vi "Dashboard Main.vi"() -> ()   [LabVIEW 2020]
uses:
  <vilib>/Utility/miscctls.llb/LVRectTypeDef.ctl
  <vilib>/Utility/miscctls.llb/LVRowAndColumnTypeDef.ctl
  <vilib>/event_ctls.llb/eventvkey.ctl
  <vilib>/Rock Robotics/WPI/DriverStation/WPI_DriverStationAllianceInfo.ctl
  <vilib>/Utility/xml.llb/Read From XML File(array).vi
  <vilib>/Utility/xml.llb/Write to XML File(string).vi
  <vilib>/Rock Robotics/Network Tables/NT Read Boolean.vi
  <vilib>/Rock Robotics/Network Tables/NT Write Boolean.vi
  <vilib>/Rock Robotics/Network Tables/NT Read Boolean Array.vi
  <vilib>/Rock Robotics/Network Tables/NT Write Boolean Array.vi
  <vilib>/Rock Robotics/Network Tables/NT Write Numeric Array.vi
  <vilib>/Rock Robotics/Network Tables/NT Read Numeric Array.vi
  <vilib>/Rock Robotics/WPI/Dashboard/WPI_DashboardLogging Global.vi
  <vilib>/Rock Robotics/Network Tables/NT Write String Array.vi
  <vilib>/vision/NI_Vision_Development_Module.lvlib
panel:
  out "Legal_Drivers":string[](array[string])
  out "Shooter_Motor_Failure_Array":bool[](array[boolean])
  out "Shooter_Overheat_Array":bool[](array[boolean])
  out "Shifter_Faults_Array":bool[](array[boolean])
  out "Drive_Overheat_Array":bool[](array[boolean])
  out "Audible_Warnings_Enabled":bool
  in  "TCP":refnum<k5>
  in  "Rec Mode":enum32{"Stop", "Record", "Playback"}(radio)
  out "Image Message":string="Timeout in Camera Communications"
  in  "Dashboard Tab":T1(tab)=enum."Setup/Auto"
  in  "CheckList":i32(listbox)
  out "Match_End":bool
  out "Auto Playbook Entry":string
  out "Drive Action":string
  out "Manipulator Action":string
  in  "Driver Profile":u16(ring) items=["N/A"]
  in  "Camera Name":string(combo)="limelight"
  in  "Camera Settings":T2={"Frame Rate"=20, "Compression"=60, "Size"=1, "DB Camera Config"=FALSE} {"Size" items=["640x480", "320x240", "160x120"]}
  in  "Autonomous Play":u16(ring) items=["N/A"]
  out "Robot Pose":cluster{dbl[], dbl[]}[](graph)
  out "Master_Caution_0":bool caption="Mode_Butterfly"
  out "Robot_is_Autonomous_0":bool caption="Mode_Butterfly"
  in  "Robot Profile":u16(ring) items=["N/A"]
  out "Robot_Code_Version":string
  in  "Default Camera Pipeline":u16(ring) items=["N/A"]
  out "Auto_Suffix":string
  in  "Refresh_Auto_Play_List":bool
  in  "Auto_Delay":dbl format="%.1f"
  in  "Warning Time (s)":dbl=30.0 format="%.1f"
  in  "Manual_Start_X":dbl=509.25 format="%.1f"
  in  "Disable_Fusion_X":bool=TRUE
  out "Robot X":dbl format="%.1f"
  out "Robot Y":dbl format="%.1f"
  in  "Manual_Start_Y":dbl=94.66 format="%.1f"
  in  "Disable_Fusion_Y":bool=TRUE
  out "Robot H":dbl format="%.1f"
  in  "Manual_Start_H":dbl format="%.1f"
  out "Distance_To_Target_Detail":dbl format="%.1f"
  in  "Field Map":u16(ring) items=["N/A"]
  in  "Push_Robot_Start":bool
  in  "Export_Robot_Pose":bool
  in  "Clear_Robot_Pose_Display":bool
  in  "Dock_Dashboard":bool
  in  "Hide_Popups":bool
  in  "Force_Human_Control":bool
  in  "Auto_Test_Mode":bool
  out "Camera_1_Fault":bool
  out "Pressure_Leak":bool
  in  "Master_Safety_Override_2":bool
  in  "Master_Safety_Override_1":bool
  out "LIDAR_Fault":bool
  out "Help Graphic":T3(plugin-control)
  in  "Manipulator_Help":bool
  out "Cowl_Position":dbl(knob) scale=0.0..1.0
  in  "Driver_Help":bool
  in  "Error_Help":bool
  out "Camera_2_Fault":bool
  out "Robot Pose 1":cluster{dbl[], dbl[]}[](graph)
  out "Drive_Train_Shifter":bool
  out "Electrical_Fault":bool
  out "Diverting_Power":bool
  out "Shooter_Power":dbl(knob) scale=0.0..1.0
  out "Kicker_Power":dbl(knob) scale=0.0..1.0
  out "CAN_Bus_Fault":bool
  out "IMU_Failure":bool
  out "Robot_is_Autonomous_1":bool caption="Mode_Butterfly"
  in  "Pre_Spin":bool
  out "LL_Valid":bool caption="Mode_Butterfly"
  in  "Clear_Jams":bool
  out "Balls_Shot":i32 format="%#.0f"
  out "Ret_Feeder_Left":bool
  out "Ret_Feeder_Right":bool
  out "Tablet_Override":bool
  out "Match Time(s)":sgl format="%#.0f"
  out "Intake_Overheat":bool
  out "Ret_Ball_Left":bool
  out "Ret_Ball_Right":bool
  out "Shooter_Motor_Failure":bool
  out "Intake_On":bool caption="Mode_Butterfly"
  out "Shooter_Overheat":bool
  out "Auto_Error":bool
  in  "Clear_Errors":bool
  out "Drive_Train_Azimuth":bool
  out "Pressure_Transducer":dbl(slide) scale=0.0..120.0
  out "Pressure_Vent":bool
  out "Shooter_RPM_Actual":dbl(slide) scale=0.0..5700.0
  out "Drive_Train_Overheat":bool
  out "Compressor_On":bool
  out "Ret_Power_Port_Right":bool
  out "Ret_Power_Port_Left":bool
  in  "Right":bool
  in  "Reticule":T4(ring)
  in  "Save":bool
  in  "Up":bool
  in  "Down":bool
  in  "Left":bool
  out "Master_Caution_1":bool caption="Mode_Butterfly"
  out "Battery_Critical":bool
  out "Battery_Voltage":dbl(slide) scale=11.0..13.0
  out "Field_Oriented":bool caption="Mode_Butterfly"
  out "Shooter_RPM_Goal":dbl(slide) scale=0.0..5700.0
  out "Slow_Loop":bool
  in  "Mode_TargetingComputer":bool
  in  "Mode_Wall":bool
  in  "Arm_Climber":bool
  in  "State_Normal":bool
  in  "State_Rotation_Control":bool
  in  "State_Climb":bool
  in  "Mode_InitiationLine":bool
  in  "Mode_CloseTrench":bool
  in  "Mode_FarTrench":bool
  in  "State_Position_Control":bool
  out "Combined Camera Feed":T3(plugin-control)
  out "High_Gear_0":bool
  out "High_Gear_1":bool
  out "High_Gear_2":bool
  out "High_Gear_3":bool
  out "Pointed_At_Target":bool caption="Mode_Butterfly"
  out "Shooter_Ready":bool caption="Mode_Butterfly"
  out "Shooter_Firing":bool caption="Mode_Butterfly"
  out "Shooter_Spinning":bool caption="Mode_Butterfly"
  out "Climber_Climbing":bool caption="Mode_Butterfly"
  out "Shooter_1_Temp":dbl
  out "Shooter_RPM_Goal_Detail":dbl
  out "Wheel_3S_Velocity":dbl format="%.1f"
  out "Wheel_3_Azimuth":dbl format="%.1f"
  out "Wheel_3S_Temp":dbl
  out "Wheel_0S_Temp":dbl
  in  "Select Auto":string(combo)="Select Autonomous ..."
  out "Camera Perf":string
  out "Control Loop Time (ms)":u32
  in  "Calibrate_Wheels":bool
  in  "Zero_Wheels":bool
  out "Wheel_0_Azimuth":dbl format="%.1f"
  out "Wheel_0S_Velocity":dbl format="%.1f"
  out "Wheel_1S_Velocity":dbl format="%.1f"
  out "Wheel_1_Azimuth":dbl format="%.1f"
  out "Wheel_1S_Temp":dbl
  out "Wheel_2S_Velocity":dbl format="%.1f"
  out "Wheel_2_Azimuth":dbl format="%.1f"
  out "Wheel_2S_Temp":dbl
  in  "Arm_Calibrate":bool
  out "Shooter_0_RPM_Actual_Detail":dbl
  out "Master_Caution_2":bool caption="Mode_Butterfly"
  out "Shooter_0_Temp":dbl
  out "Shooter_1_RPM_Actual_Detail":dbl
  out "Out_Of_Range":bool
  in  "New_Shooter_Setpoint (rpm)":dbl=3000.0 min=0.0 max=5700.0 step=100.0
  out "Kicker_RPM_Actual_Detail":dbl
  out "Kicker_RPM_Goal_Detail":dbl
  out "Kicker_Temp":dbl
  out "Intake_Temp":dbl
  in  "Actuator Testing":u16(ring) items=["N/A"]
  in  "Test_Actuator_Value":dbl step=0.1 format="%.2f"
  in  "Calibrate_Joysticks":bool
  in  "Arm_Calibrate_Joysticks":bool
  out "Robot_is_Autonomous_2":bool caption="Mode_Butterfly"
  in  "Test_Actuator_Period":dbl min=0.0 step=1.0 format="%.2f"
  out "Pose Loop Time (ms)":u32
  in  "Mute_Audible_Warnings":bool
  out "Combined Error String":string
  out "LIDAR_Distance_To_Target":dbl format="%.1f"
  out "Beam_Break_Raw":i32
  out "Wheel_0_Shifter_State":string
  out "Wheel_1_Shifter_State":string
  out "Wheel_3_Shifter_State":string
  out "Wheel_2_Shifter_State":string
  out "Azimuth_Error_Array":bool[](array[boolean])
  out "Selected_Shooter_Setpoint_Value (rpm)":dbl
  in  "Apply_New_Shooter_Setpoint":bool
  in  "Selected_Shooter_Setpoint_Index":u16(ring) items=["N/A"]
  in  "Auto_Target_Override":bool
  in  "Field_Oriented_Override":bool
  in  "Camera_Override":bool
  in  "Super_Test_Mode":bool
  out "Current_Driver_Profile_Setpoints":T5={"Strafe Deadband"=0.08, "Strafe Scaling"=2.0, "Strafe Maximum"=0.5, "Rotation Deadband"=0.15, "Rotation Scaling"=2.5, "Rotation Maximum"=0.5} {"Rotation Maximum" min=0.3 max=1.0 scale=0.3..1.0; "Rotation Scaling" min=1.0 max=4.0 scale=1.0..4.0; "Rotation Deadband" min=0.0 max=0.25 scale=0.0..0.25; "Strafe Maximum" min=0.3 max=1.0 scale=0.3..1.0; "Strafe Scaling" min=1.0 max=4.0 scale=1.0..4.0; "Strafe Deadband" min=0.0 max=0.25 scale=0.0..0.25}
  in  "New_Driver_Profile_Setpoints":T6={"Strafe Deadband"=0.08, "Strafe Scaling"=2.0, "Strafe Max"=0.5, "Rotate Deadband"=0.15, "Rotate Scaling"=2.5, "Rotate Max"=0.5} {"Rotate Max" min=0.3 max=1.0 format="%.2g"; "Rotate Scaling" min=1.0 max=4.0 format="%.2g"; "Rotate Deadband" min=0.0 max=0.25 format="%.2g"; "Strafe Max" min=0.3 max=1.0 format="%.2g"; "Strafe Scaling" min=1.0 max=4.0 format="%.2g"; "Strafe Deadband" min=0.0 max=0.25 format="%.2g"}
  in  "Apply_Driver_Profile_Setpoints":bool
  out "Current_Driver_Profile":string
  out "NT Connection":bool
  out "Mode":T7(ring)=enum."Auto Disabled"
  in  "Test Slider":dbl(slide) scale=0.0..100.0 scale format="%#_3g"
  in  "On/Off":bool caption="Solenoid"
  in  "Test Name":u16(ring) items=["Select the test to run..."]
  in  "Test Tree":string(tree)
  in  "Motor":cluster{"Value":dbl, "Enable":bool} {"Value" scale=-1.0..1.0 scale format="%#_3g"}
  out "Progress":T8 {"Test Progress" scale=0.0..100.0}
  in  "Rev/Fwd":cluster{"Forward":bool, "Reverse":bool}
  in  "Test Ring":u16(ring) items=["Monochrome", "Color"]
  out "Cmd Status":string
  in  "Execute Command":bool
  in  "Command Params":string[][](table)
  in  "Command Selection":i32(listbox)
  out "Tree":string(tree)
  out "Background":bool
  # "2022 Dashboard v1.0-dev"
  # "Auto Delay (s)"
  # "Auto Play Suffix"
  # "Robot X (in)"
  # "Endgame Alert (s)"
  # "Robot Y (in)"
  # "Robot H (deg)"
  # "Range to Target (in)"
  # "Undock Dashboard"
  # "Hide\nPopups"
  # "Auto Test\nMode"
  # "Force\nHuman"
  # "Drive Action"
  # "Dock Dashboard"
  # "Dynamic Popups"
  # "Auto Real Mode"
  # "Robot\nDecides"
  # "Manipulator Action"
  # "C"
  # "K"
  # "S"
  # "11"
  # "13"
  # "0"
  # "120"
  # "0"
  # "1"
  # "2"
  # "3"
  # "Drivebase Subsytem"
  # "Shooter Subsystem"
  # "Calibrate Joysticks"
  # "Control"
  # "Pose"
  # "Driver Profile Setpoints"
  # "LIDAR\nDistance (in)"
  # "Latency\n(ms)"
  # "Shoot 0"
  # "Shoot 1"
  # "Kicker"
  # "Module 1"
  # "Module 0"
  # "Azimuth (deg)"
  # "Speed Goal (rpm)"
  # "Temp (C)"
  # "Beam Break"
  # "Speed Actual (rpm)"
  # "Auto Target Override"
  # "Robot-Oriented"
  # "Camera Override"
  # "Super Test Mode"
  # "Velocity (ft/s)"
  # "Temp (C)"
  # "Shifter State"
  # "Setpoints"
  # "Module 2"
  # "Module 3"
  # "Azimuth (deg)"
  # "Normal \nAuto Target"
  # "Field-Oriented"
  # "Normal Camera"
  # "Normal Operation"
  # "Temp (C)"
  # "(rpm)"
  # "Velocity (ft/s)"
  # "Ball Handling Subsystems"
  # "Shifter State"
  # "Intake"
  # "p: power [-1,1]\nb: boolean {0,1}\nr: rpm (-inf,+inf)\na: angle [0,+inf)"
  # "Amplitude"
  # "Calibrate Wheels"
  # "Temp (C)"
  # "Period (s)"
  # "0"
  # "0.25"
  # "1"
  # "4"
  # "0.3"
  # "1"
  # "0"
  # "0.25"
  # "1"
  # "4"
  # "0.3"
  # "1"
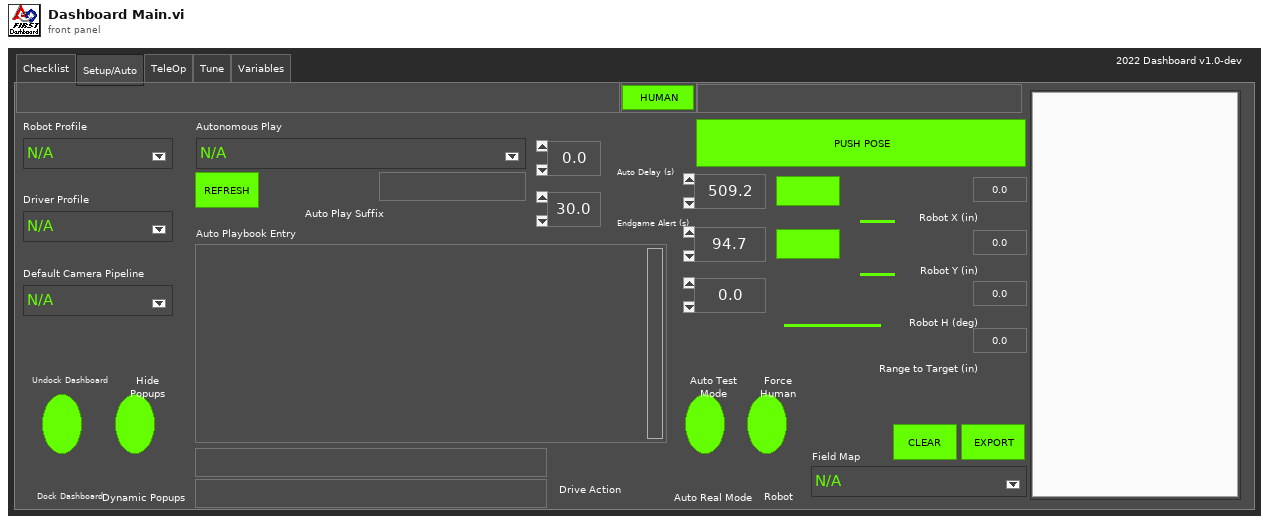
[diagram p1: front panel]
types:
  T1 = enum32{"Checklist", "Setup/Auto", "TeleOp", "Tune", "NT", "Test", "Commands", "Variables"}
  T2 = cluster{"Frame Rate":i32, "Compression":i32, "Size":u16, "DB Camera Config":bool}
  T3 = typedef "IMAQ Image.ctl" = refnum<image>
  T4 = enum16{"Power Port Left", "Power Port Right", "Ball Left", "Ball Right", "Feeder Left", "Feeder Right"}
  T5 = cluster{"Strafe Deadband":dbl, "Strafe Scaling":dbl, "Strafe Maximum":dbl, "Rotation Deadband":dbl, "Rotation Scaling":dbl, "Rotation Maximum":dbl}
  T6 = cluster{"Strafe Deadband":dbl, "Strafe Scaling":dbl, "Strafe Max":dbl, "Rotate Deadband":dbl, "Rotate Scaling":dbl, "Rotate Max":dbl}
  T7 = enum8{"Tele-Op Disabled", "Tele-Op Enabled", "Auto Disabled", "Auto Enabled", "Test Disabled", "Test Enabled", "Disconnected", "No Code", "E-Stop"}
  T8 = cluster{"Test Progress":u8, "Test Progress Text":string}
  T9 = cluster{"Save Path":path, "Interval (s)":dbl, "Keep":i32}
  T10 = enum32{"Drive", "Camera", "Basic", "Custom", "Test", "Commands", "Checklist", "Variables"}
  T11 = cluster{"IDs":cluster{"RPC field ID":u16, "Unique ID":u16}, "String":string}
  T12 = typedef "Image Type" = u32
  T13 = cluster{"Ret_Power_Port_Left":refnum<vi>, "Ret_Power_Port_Right":refnum<vi>, "Ret_Ball_Left":refnum<vi>, "Ret_Ball_Right":refnum<vi>, "Ret_Feeder_Left":refnum<vi>, "Ret_Feeder_Right":refnum<vi>}
  T14 = cluster{"Camera Name":string, string, "Saved DB Images Info":cluster{"Save Path":path, "Interval (s)":dbl, "Keep":i32}}
  T15 = typedef "WPI_DriverStationAllianceInfo.ctl" = enum16{"Red", "Blue", "Invalid"}
  T16 = enum8{"Enabled", "Disabled", "Disabled and Grayed Out"}
  T17 = cluster{"Error Strings":string, "Disable Counts":cluster{u16, u16}, "Rail Faults":cluster{u16, u16, u16}, "Robot IP":string, "DB Mode":u8, "Event Info":cluster{"Name":string, "Type":u8, "Number":u16, "Replay":u8}}
  T18 = cluster{"Storage":cluster{"Disk Free":u64, "RAM Block":u32, "RAM free":u32}, "CPU Utilization":cluster{"CPU % ISR":sgl, "CPU % Time Crit":sgl, "CPU % Timed Str":sgl, "CPU % High":sgl, "CPU % Above":sgl, "CPU % Normal":sgl, "CPU % Low":sgl}, "CAN":cluster{"% Bus Utilization":sgl, "Bus Off Cnt":u32, "TX_FIFO Full Cnt":u32, "Receive Error Cnt":u8, "Transmit Error Cnt":u8}, "HID":cluster{"HID Outputs":u32, "Rumble Low":u16, "Rumble High":u16}[]}
  T19 = cluster{"Status bits":cluster{"Test Mode":bool, "Autonomous":bool, "Enabled":bool, "Code Start":bool, "Brownout":bool, "Reserved 2":bool, "Reserved 3":bool, "E-Stop":bool}, "Code Trace":cluster{"Disabled":bool, "TeleOp":bool, "Auto":bool, "Test":bool}, "Controller Type":enum16{"unknown", "cRIO", "roboRio"}, "Code?":enum16{"unknown", "noCode", "code"}, "Battery V":dbl}
  T20 = cluster{"Control Bits":cluster{"TestMode":bool, "Autonomous":bool, "Enabled":bool, "FMS Present":bool, bool, bool, bool, "E-Stop":bool}, "Team Station ":u8, "Countdown":sgl, "Joystick Values":cluster{"Axes":dbl[], "Buttons":bool[], "POVs":i16[]}[]}
  T21 = typedef "imagedata.ctl" = cluster{"image type":i32, "image depth":i32, "image":u8[], "mask":u8[], "colors":u32[], "Rectangle":cluster{"left":i16, "top":i16, "right":i16, "bottom":i16}}
  T22 = cluster{"Numeric Array[0]":dbl, "Numeric Array[1]":dbl, "Numeric Array[2]":dbl, "Numeric Array[3]":dbl, "Numeric Array[4]":dbl, "Numeric Array[5]":dbl}
  T23 = cluster{bool, "Super_Test_Mode":bool, "Slow_Loop":bool, "Drive_Train_Overheat":bool, "Pressure_Vent":bool, "Drive_Train_Azimuth":bool, "Arm_Calibrate":bool, "Auto_Error":bool, "Auto_Test_Mode":bool, "Shooter_Overheat":bool, "Shooter_Motor_Failure":bool, "Intake_Overheat":bool, bool, "IMU_Failure":bool, "Electrical_Fault":bool, "Arm_Calibrate_Joysticks":bool, "CAN_Bus_Fault":bool, "Drive_Train_Shifter":bool, "Battery_Critical":bool}
  T24 = cluster{"Operation":enum16{"Update", "Clear"}, "Color Box":u32}[]
  T25 = typedef "eventvkey.ctl" = enum16{"ASCII", "Enter", "Return", "Shift", "Ctrl", "Alt", "Cmd", "Opt", "Caps", "NumLock", "Clear", "Break", "Up", "Down", "Left", "Right", "Insert", "Delete", "Home", "End", "PageUp", "PageDown", "Escape", "Help", "Pause", "ScrollLock", "F1", "F2", "F3", "F4", "F5", "F6", "F7", "F8", "F9", "F10", "F11", "F12", "F13", "F14", "F15", "F16", "F17", "F18", "F19", "F20", "F21", "F22", "F23", "F24", "Play", "VolumeUp", "VolumeDown", "Mute", "Two Byte Char"}
  T26 = cluster{"Image Size":bool, "Image Type":bool, "Pixel Value":bool, "ROI Information":bool, "Zoom Factor":bool}
  T27 = cluster{"Operation":enum16{"Update", "Clear"}, "Color Box":u32}
  T28 = typedef "LVRowAndColumnTypeDef.ctl" = cluster{"Row":i32, "Column":i32}
  T29 = cluster{"Shift":bool, "Ctrl":bool, "Alt":bool, "Cmd":bool, "Opt":bool}
  T30 = cluster{string, "Drive_Train_Overheat":bool, dbl}
  T31 = cluster{string, "Shooter_Motor_Failure":bool, dbl}
  T32 = cluster{string, "Arm_Calibrate_Joysticks":bool, dbl}
  T33 = cluster{string, "Drive_Train_Shifter":bool, dbl}[]
  T34 = typedef "LVRectTypeDef.ctl" = cluster{"Left":i16, "Top":i16, "Right":i16, "Bottom":i16}
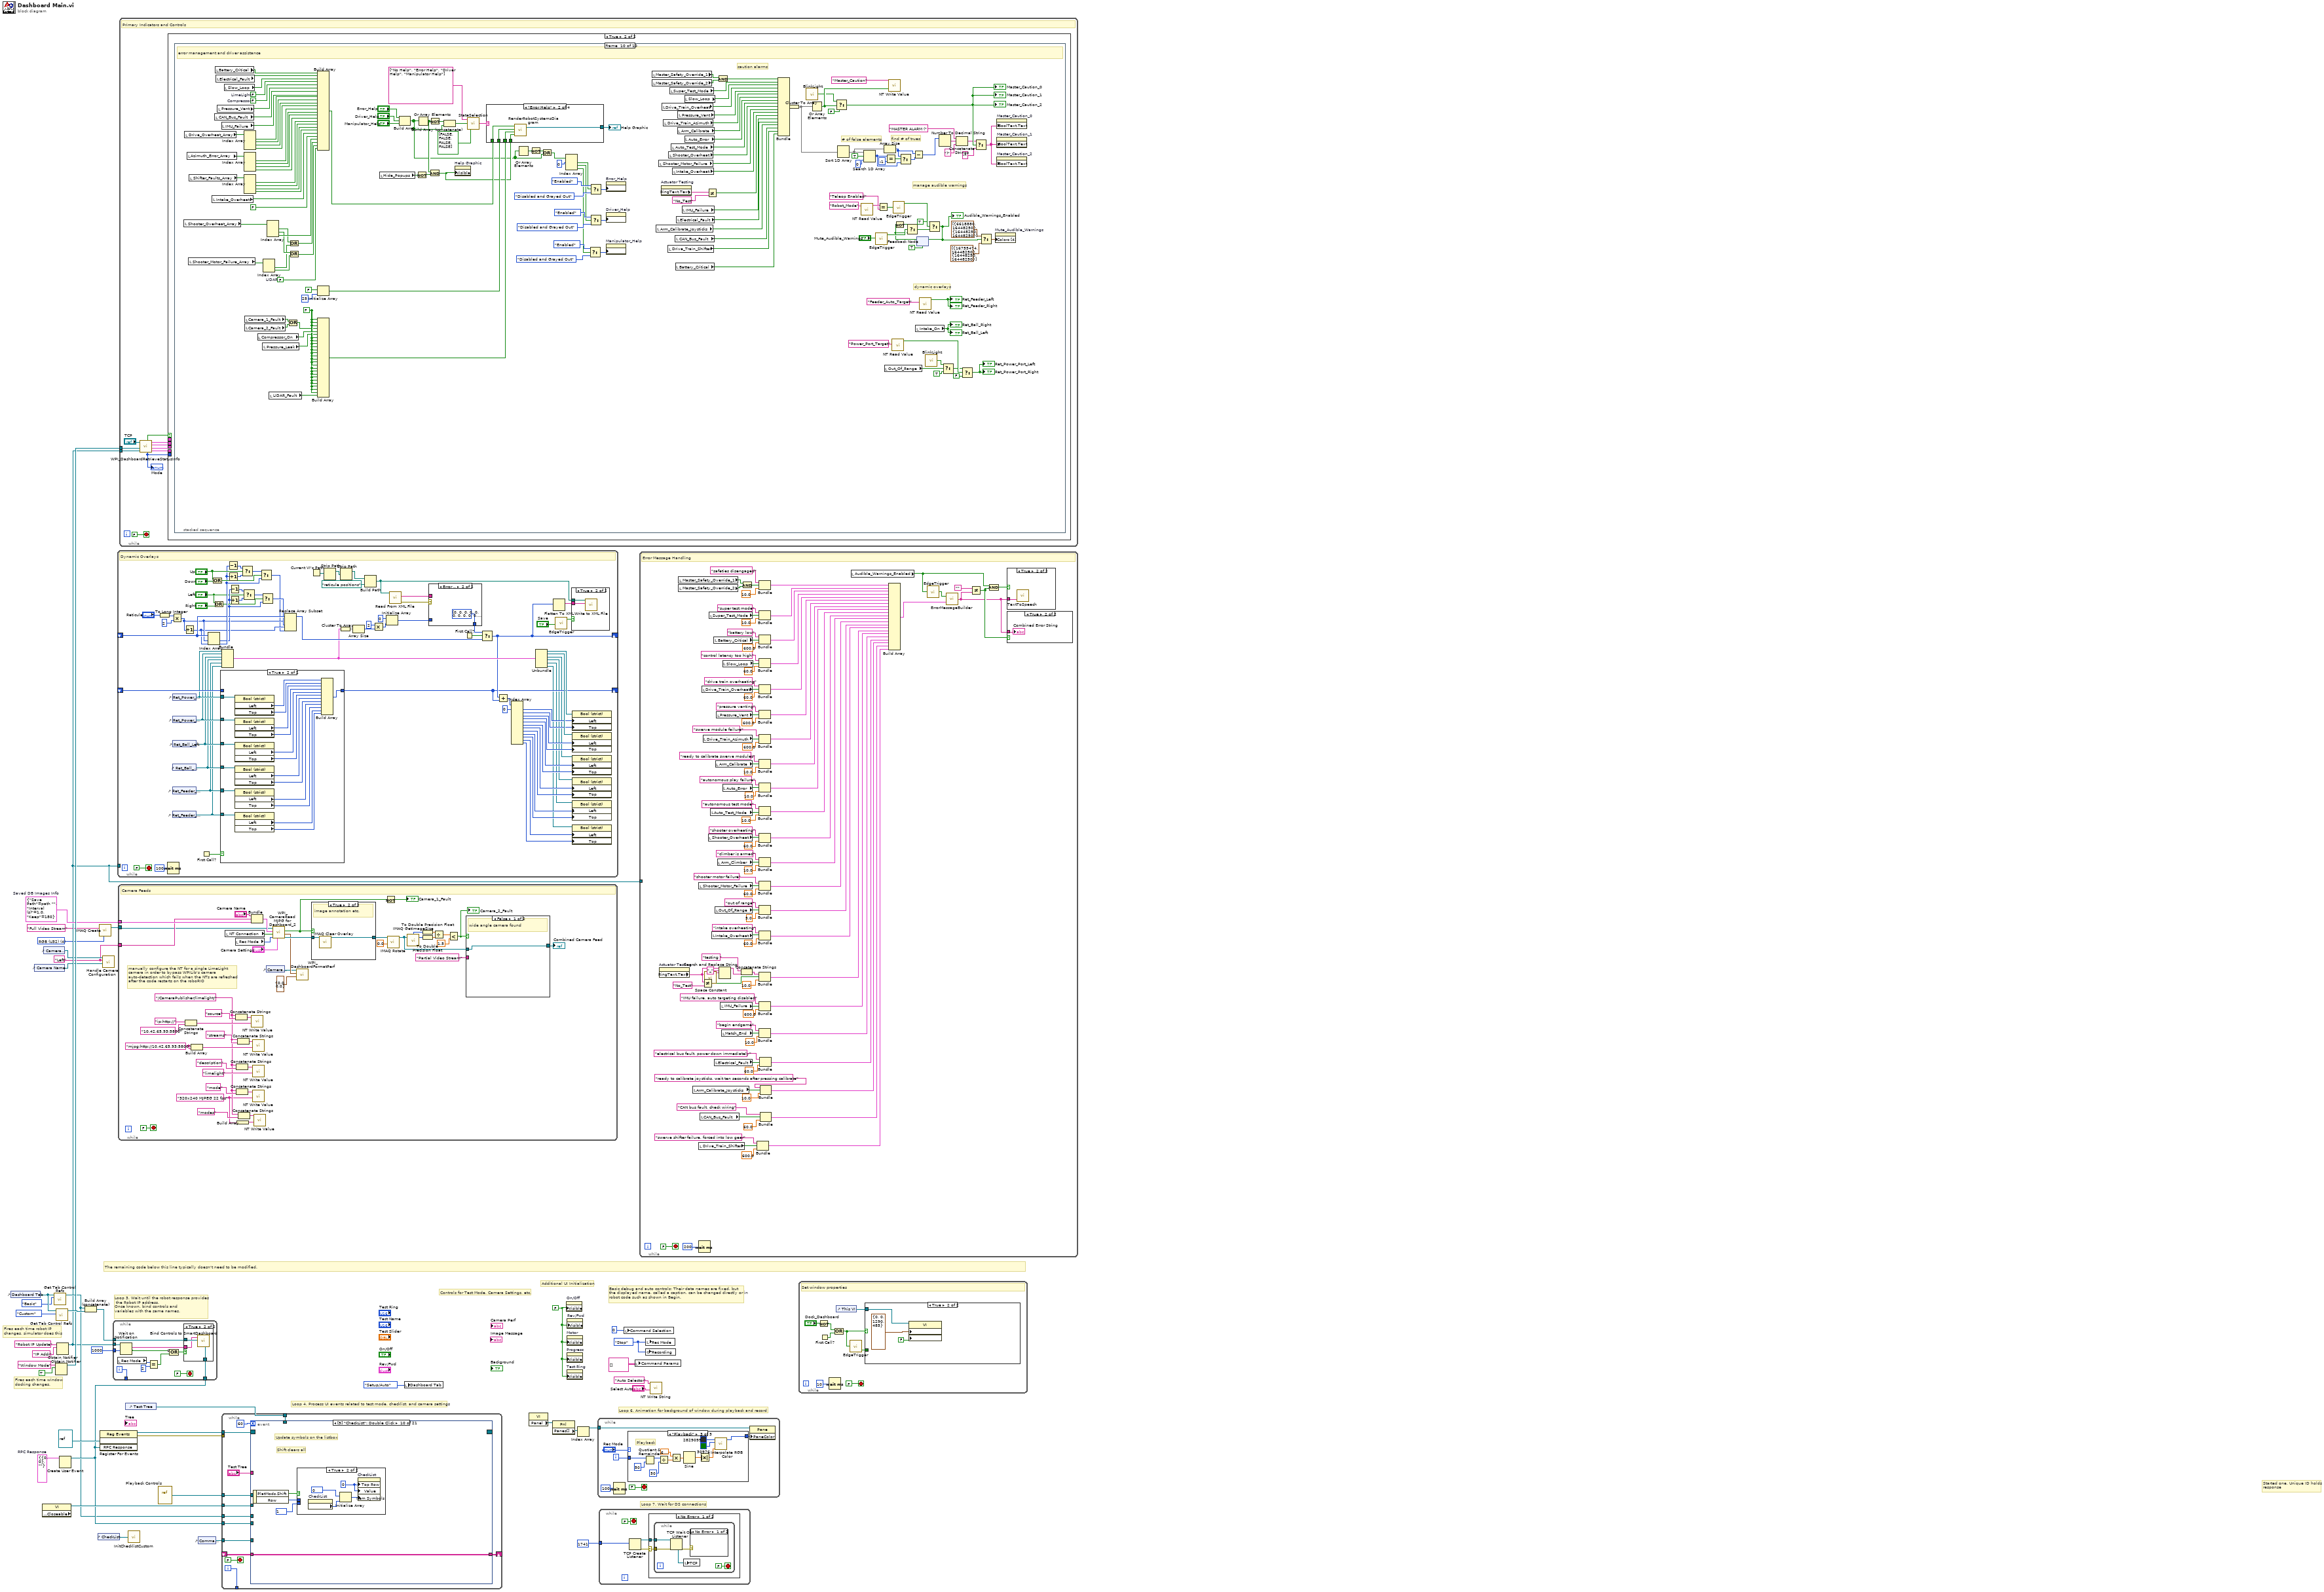
[diagram p0: block diagram]
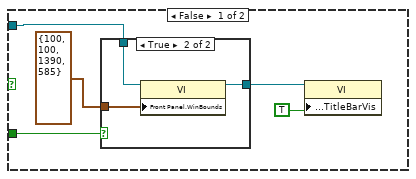
[diagram p2: hidden frame]
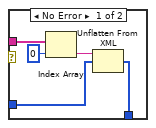
[diagram p6: hidden frame]
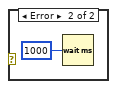
[diagram p9: hidden frame]
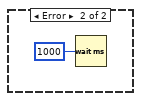
[diagram p10: hidden frame]
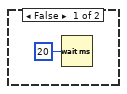
[diagram p11: hidden frame]
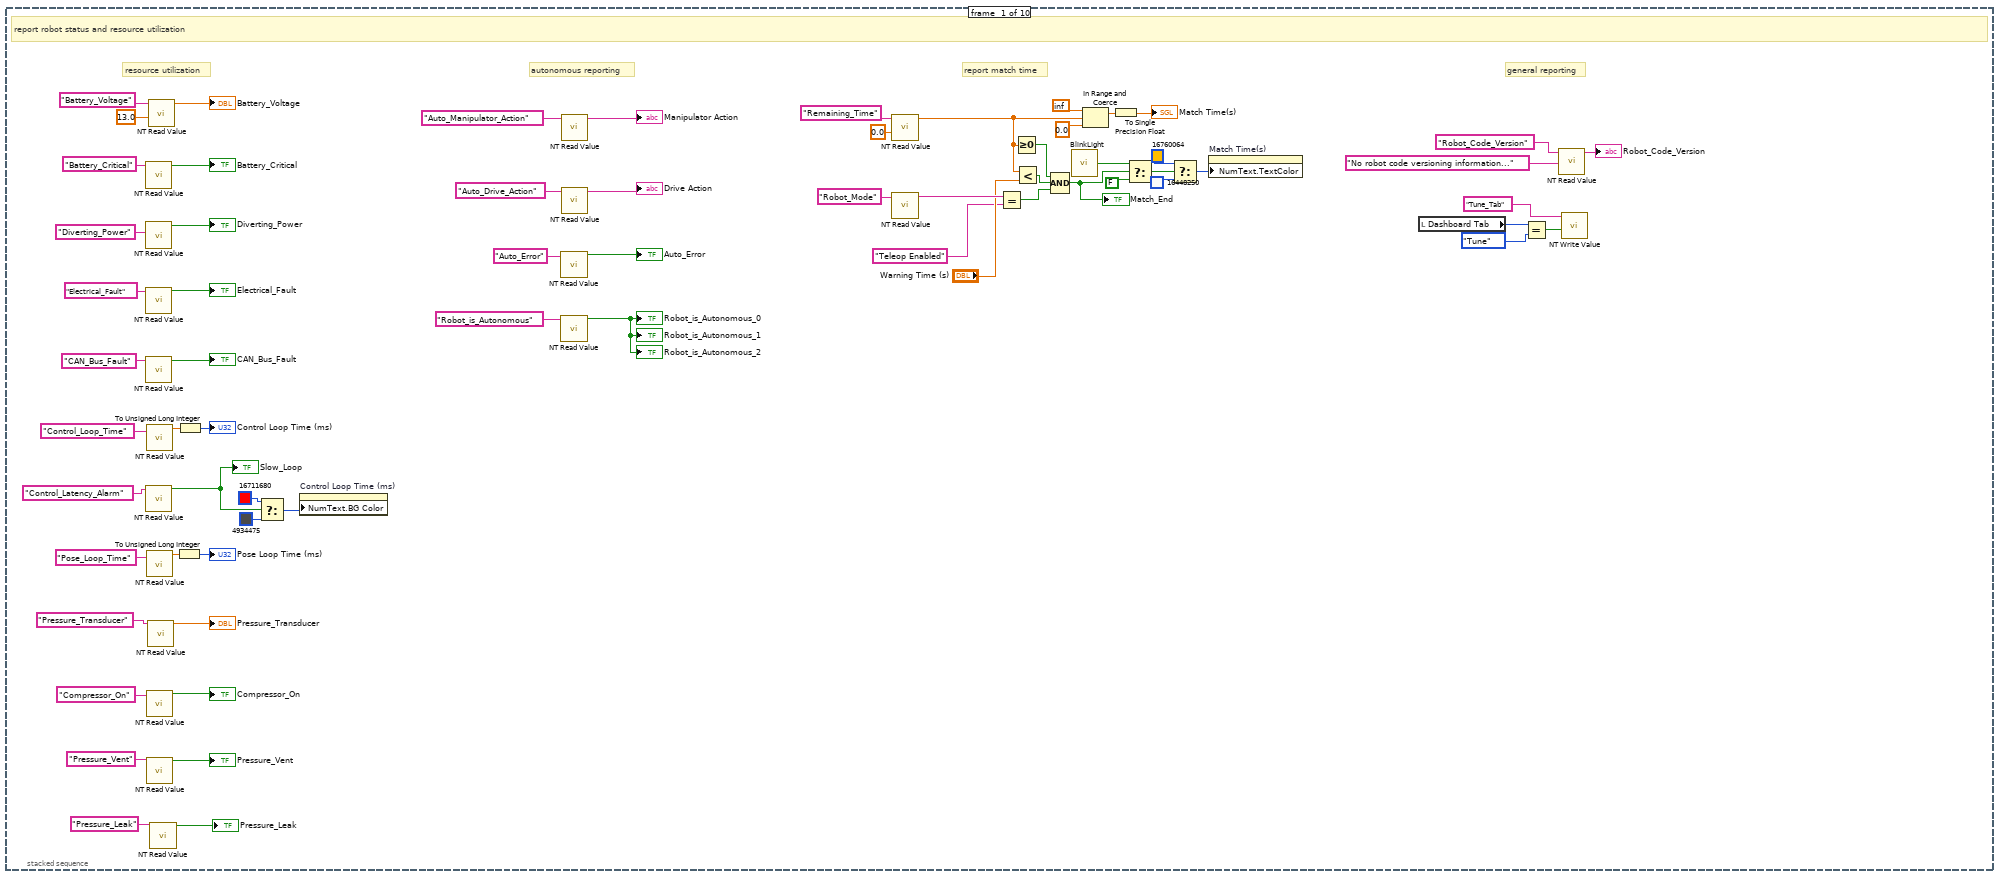
[diagram p12: hidden frame]
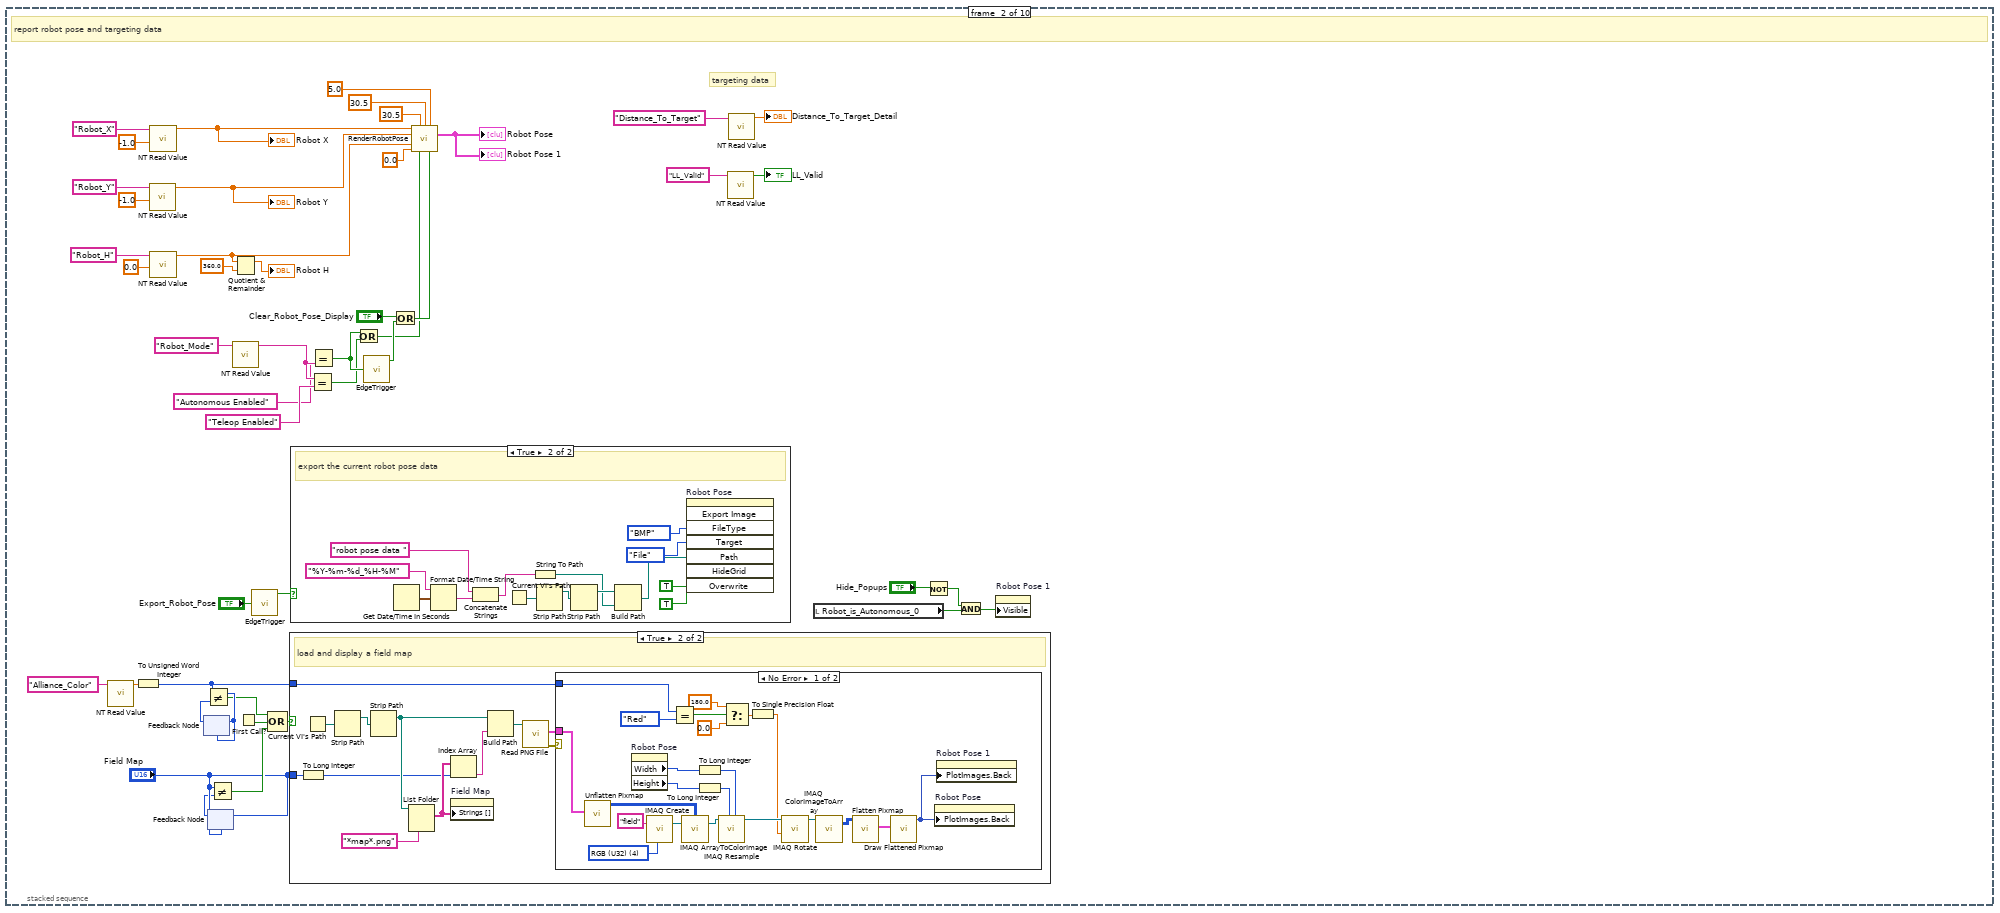
[diagram p13: hidden frame]
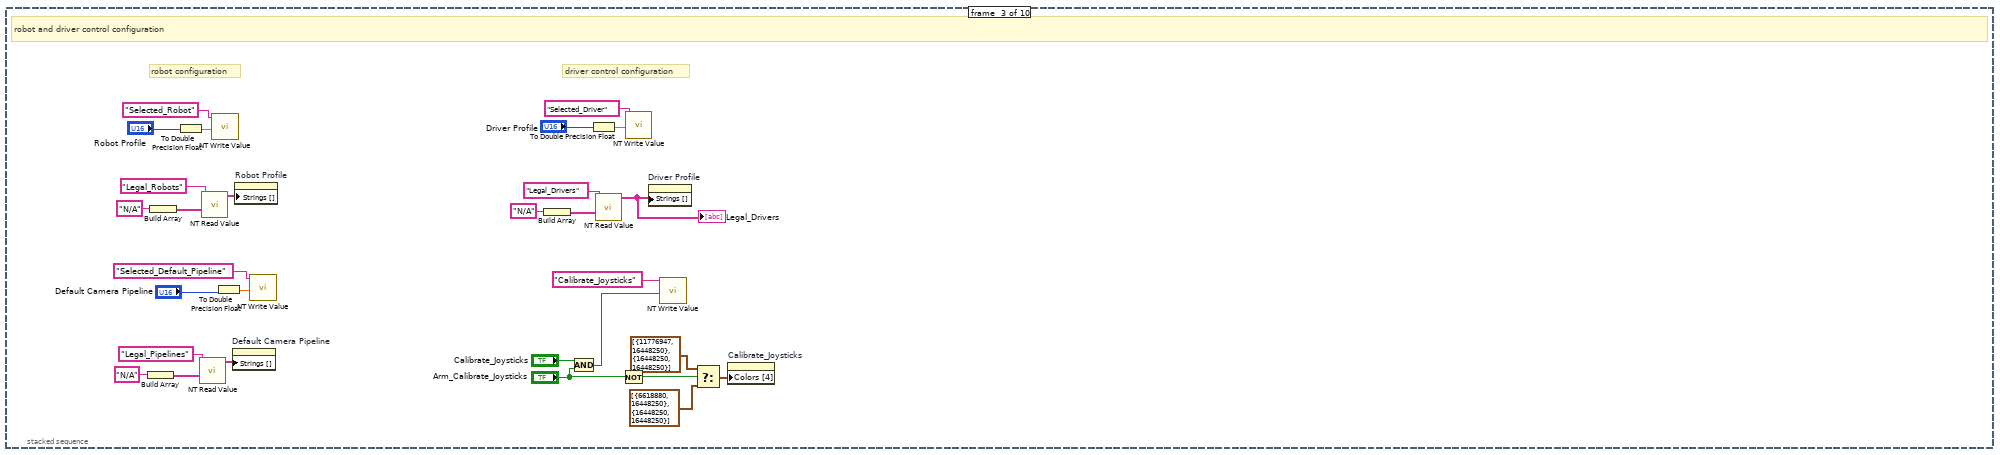
[diagram p17: hidden frame]
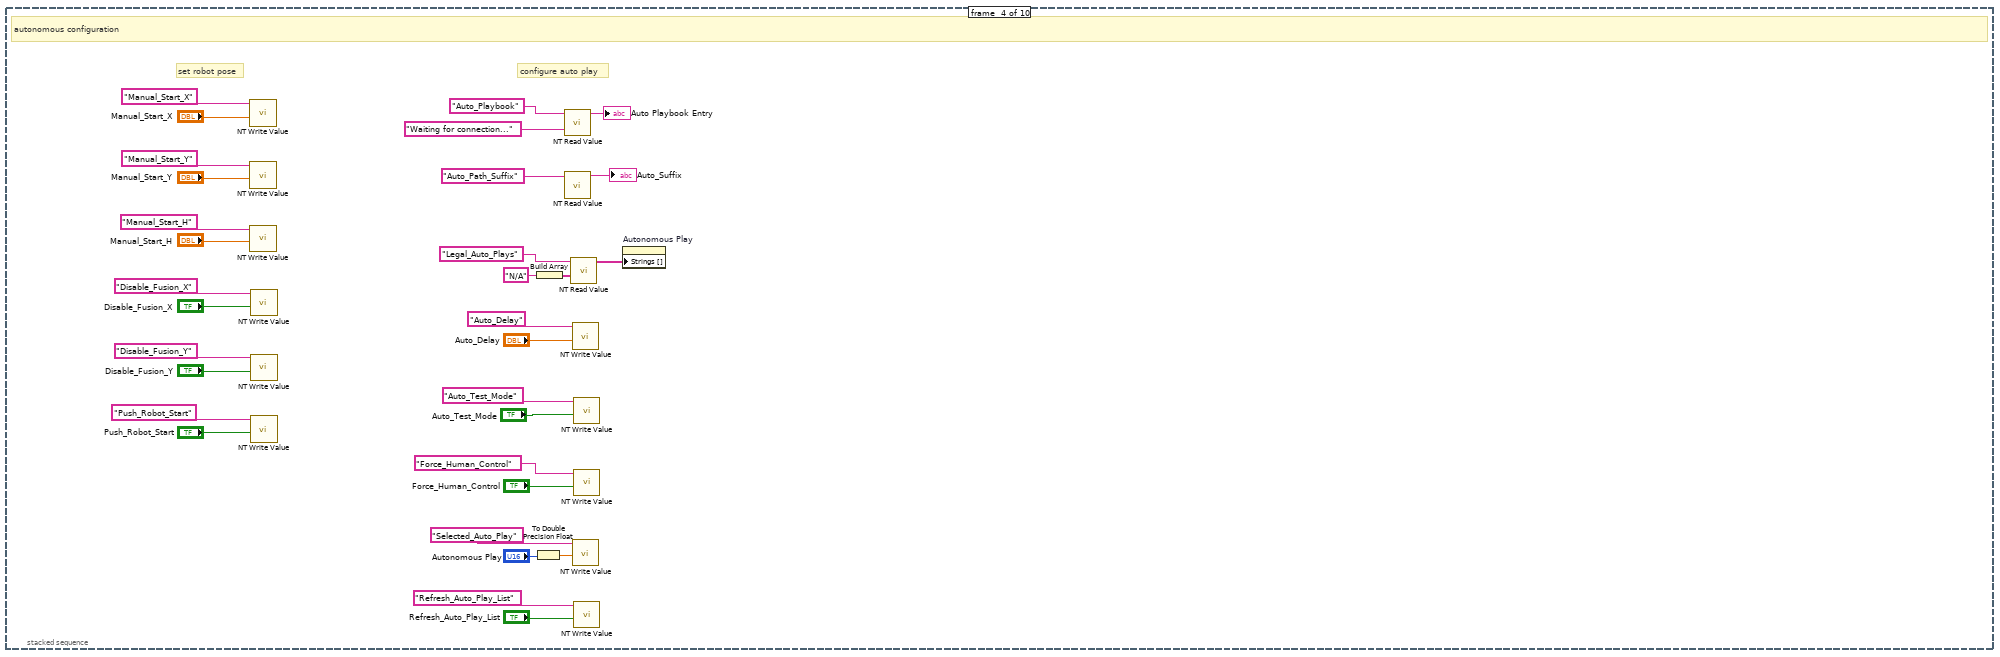
[diagram p18: hidden frame]
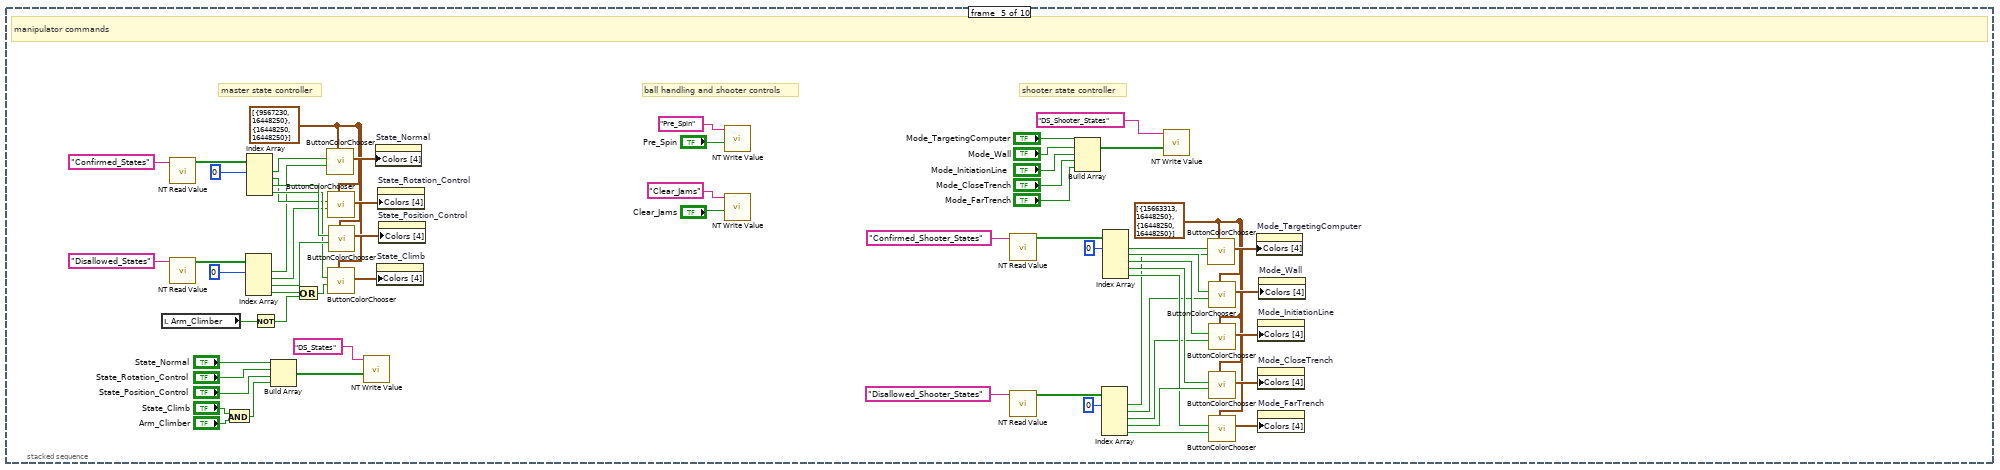
[diagram p19: hidden frame]
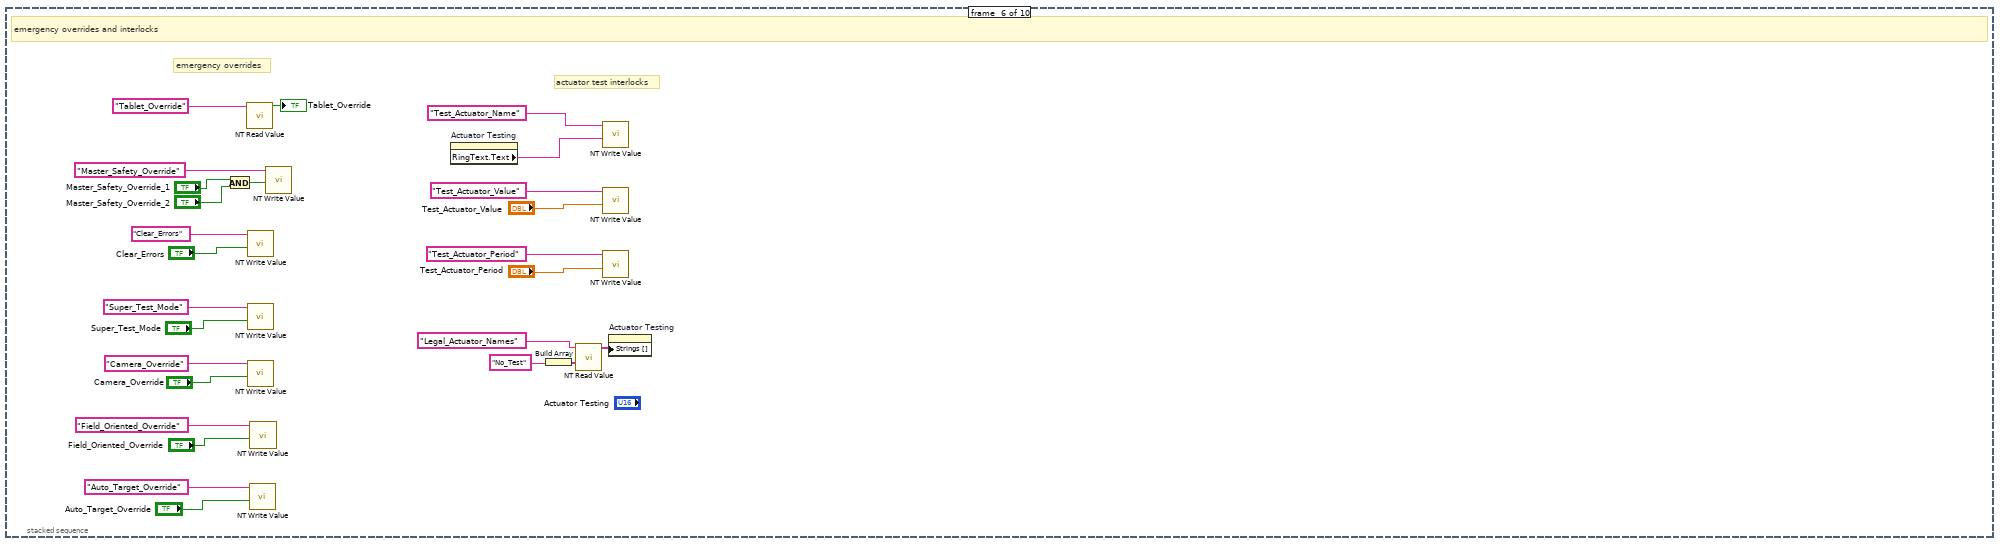
[diagram p20: hidden frame]
diagram:
  w9 = T9 {"Save Path"=path "", "Interval (s)"=1.0, "Keep"=180}  # Saved DB Images Info
  w6 = "Left"
  w19 = T11 {"IDs"={"RPC field ID"=0, "Unique ID"=0}, "String"=""}  # RPC Response
  w28 = enum32{"Stop", "Record", "Playback"}."Stop" ("Rec Mode")
  w23 = FALSE ("Visible")
  w3 = T12 4 items=["Grayscale (U8)", "Grayscale (I16)", "Grayscale (SGL)", "Complex (CSG)", "RGB (U32)", "HSL (U32)", "RGB (U64)"] ("Image Type")
  # "Started one, Unique ID holds\nresponse"
  # "Loop 7. Wait for DS connections"
  # "Basic debug and auto controls: Their data names are fixed, but\nthe displayed name, called a caption, can be changed directly or in\nrobot code such as shown in Begin."
  # "Controls for Test Mode, Camera Settings, etc."
  # "Additional UI Initialization"
  # "Loop 6. Animation for background of window during playback and record"
  # "Fires each time robot IP\nchanges, simulator does this"
  # "Fires each time window\ndocking changes."
  # "The remaining code below this line typically doesn't need to be modified."
  # "Loop 4. Process UI events related to test mode, checklist, and camera settings"
  # "Loop 3. Wait until the robot response provides\n the Robot IP address.\nOnce known, bind controls and\nvariables with the same names."
  n1 = control-ref of="Dashboard Tab"() -> (w26:refnum<vi>)
  n2 = control-ref of="Camera Name"() -> (w5:refnum<vi>)
  n3 = property class="VI" props=["Front Panel.Closeable"]() -> (reference out=w27:refnum<vi>)  [unwired: 2 in, 2 out]
  n4 = control-ref of="Camera Settings"() -> (w7:refnum<vi>)
  n5 = call <vilib>:"Get Tab Control Refs.vi"("Page Index"=T10."Basic" ("Dashboard Tab"), "TabControl in"=w26) -> ("ControlsOnPage"=w14:refnum<vi>[])  [unwired: 9 in]
  n6 = Obtain Notifier(name (unnamed)="Window Mode", notification data type=TRUE) -> (notifier out=w22:refnum<notifier>)  [unwired: 2 in, 2 out]
  n7 = call <vilib>:"Get Tab Control Refs.vi"("Page Index"=T10."Custom" ("Dashboard Tab"), "TabControl in"=w26) -> ("ControlsOnPage"=w25:refnum<vi>[])  [unwired: 9 in]
  n8 = Obtain Notifier(name (unnamed)="Robot IP Update", notification data type="IP Addr" ("name (unnamed)")) -> (notifier out=w8:refnum<notifier>)  [unwired: 2 in, 2 out]
  n9 = Create User Event(user event datatype=w19) -> (user event=w16:refnum<user-event>)  [unwired: 1 in, 1 out]
  n10 = Build Array (concatenate)(w14, w25) -> (w24:refnum<vi>[])
  n11 = control-ref of="CheckList"() -> (w1:refnum<vi>)
  n12 = call "IMAQ Create"("Image Name"="Full Video Stream", "Image Type"=w3) -> ("New Image"=w2:T3)  [unwired: 2 in, 2 out]
  n13 = register-events(refnum<vi> refnum, w16) -> (reference out=w32:refnum<event-registration>, error out=w31:errorcluster)  [unwired: 2 in]
  n14 = call "Handle Camera Configuration.vi"("CameraNameRef"=w5, "Display Name"=w6, "ClusterRef"=w7) -> ()  [unwired: 9 in]
  n15 = while {
    tunnel: w24 -> [w53]
    tunnel: w8 -> [w51]
    tunnel: [w49] -> _
    tunnel: u32 1000 ("milliseconds to wait") -> [w48]
    tunnel: w16 -> [w42]
    i -> [w49]
    stop <- FALSE stop-if-true
    n16 = local read "Rec Mode"() -> (w44:enum32{"Stop", "Record", "Playback"})
    n17 = Wait on Notification(notifier=w51, timeout in ms (-1)=w48) -> (notification=w50:string, timed out?=w46:bool)  [unwired: 2 in, 2 out]
    n18 = Equal?(x=w44, y=u16 2 ("Rec Mode")) -> (x = y?=w45:bool)
    n19 = Compound Arithmetic op=OR(invert w46, w45) -> (w47:bool)
    n20 = case shown="True" w47 {
      tunnel: w53 -> [_ w56]
      tunnel: w50 -> [_ w55]
      tunnel: w42 -> [_ w54]
      frame False {
      }
      frame True {
        n21 = call <vilib>:"Bind Controls to SmartDashboard.vi"("RPC ref"=w54, "Bound Control Refs"=w56, "Server IP Address"=w55) -> ()  [unwired: 9 in]
      }
    }
  }
  n22 = while {
    shift-right: [w75] -> _
    shift-left: _ -> [w128]
    shift-right: [w76] -> _
    shift-left: _ -> [w118]
    tunnel: w8 -> [_]
    stop <- FALSE stop-if-true
    # "Dynamic Overlays"
    n23 = To Long Integer(number="Reticule") -> (32bit integer=w109:i32)
    n24 = Wait (ms)(milliseconds to wait=u32 100) -> ()  [unwired: 1 out]
    n25 = Multiply(x=w109, y=2) -> (x*y=w108:i32)
    n26 = control-ref of="Ret_Power_Port_Left"() -> (w89:refnum<vi>)
    n27 = control-ref of="Ret_Power_Port_Right"() -> (w88:refnum<vi>)
    n28 = control-ref of="Ret_Ball_Left"() -> (w74:refnum<vi>)
    n29 = control-ref of="Ret_Ball_Right"() -> (w73:refnum<vi>)
    n30 = control-ref of="Ret_Feeder_Left"() -> (w62:refnum<vi>)
    n31 = control-ref of="Ret_Feeder_Right"() -> (w61:refnum<vi>)
    n32 = Increment(x=w108) -> (x+1=w95:i32)
    n33 = First Call?() -> (First Call?: T/F=w98:bool)
    n34 = Index Array(array=w118, index #1=w108, index #2=w95) -> (element #1=w112:i32, element #2=w120:i32)
    n35 = Or(x="Up", y="Down") -> (x .or. y?=w124:bool)
    n36 = Or(x="Left", y="Right") -> (x .or. y?=w114:bool)
    n37 = case shown="True" w98 {
      tunnel: [w139 w158] -> w75
      tunnel: w128 -> [w139 _]
      tunnel: w89 -> [_ w157]
      tunnel: w88 -> [_ w156]
      tunnel: w74 -> [_ w147]
      tunnel: w73 -> [_ w146]
      tunnel: w62 -> [_ w141]
      tunnel: w61 -> [_ w140]
      frame False {
      }
      frame True {
        n38 = property class="Bool (strict)"(reference=w157) -> ("Left"=w155:i32, "Top"=w154:i32)  [unwired: 1 in, 2 out]
        n39 = property class="Bool (strict)"(reference=w156) -> ("Left"=w153:i32, "Top"=w152:i32)  [unwired: 1 in, 2 out]
        n40 = property class="Bool (strict)"(reference=w147) -> ("Left"=w151:i32, "Top"=w150:i32)  [unwired: 1 in, 2 out]
        n41 = property class="Bool (strict)"(reference=w146) -> ("Left"=w149:i32, "Top"=w148:i32)  [unwired: 1 in, 2 out]
        n42 = property class="Bool (strict)"(reference=w141) -> ("Left"=w145:i32, "Top"=w144:i32)  [unwired: 1 in, 2 out]
        n43 = property class="Bool (strict)"(reference=w140) -> ("Left"=w143:i32, "Top"=w142:i32)  [unwired: 1 in, 2 out]
        n44 = Build Array(w155, w154, w153, w152, w151, w150, w149, w148, w145, w144, w143, w142) -> (w158:i32[])
      }
    }
    n45 = Bundle("Ret_Power_Port_Left"=w89, "Ret_Power_Port_Right"=w88, "Ret_Ball_Left"=w74, "Ret_Ball_Right"=w73, "Ret_Feeder_Left"=w62, "Ret_Feeder_Right"=w61) -> (w80:T13)  [unwired: 1 in]
    n46 = Decrement(x=w120) -> (x-1=w127:i32)
    n47 = Increment(x=w120) -> (x+1=w126:i32)
    n48 = Decrement(x=w112) -> (x-1=w117:i32)
    n49 = Increment(x=w112) -> (x+1=w116:i32)
    n50 = Select(t=w127, s="Up", f=w126) -> (s? t:f=w125:i32)
    n51 = Select(t=w117, s="Left", f=w116) -> (s? t:f=w115:i32)
    n52 = Select(t=w125, s=w124, f=w120) -> (s? t:f=w94:i32)
    n53 = Select(t=w115, s=w114, f=w112) -> (s? t:f=w113:i32)
    n54 = Replace Array Subset(array=w118, new element #1=w113, index #1=w108, new element #2=w94, index #2=w95) -> (w93:i32[])
    n55 = Current VI's Path() -> (path=w104:path)
    n56 = Strip Path(path=w104) -> (stripped path=w103:path)  [unwired: 1 out]
    n57 = Cluster To Array(cluster=w80) -> (array=w92:refnum<vi>[])
    n58 = Strip Path(path=w103) -> (stripped path=w102:path)  [unwired: 1 out]
    n59 = Array Size(array=w92) -> (size(s)=w91:i32)
    n60 = Build Path(base path=w102, name or relative path=path "reticule positions" ("XML File Path")) -> (appended path=w101:path)
    n61 = Multiply(x=2 ("dimension size"), y=w91) -> (x*y=w97:i32)
    n62 = Initialize Array(0, w97) -> (w87:i32[])
    n63 = call-poly <vilib>:"Read From XML File.vi"("XML File Path"=w101) -> ("error out"=w79:errorcluster, "XML Elements"=w100:string[])  [unwired: 8 in, 1 out]
    n64 = case shown="Error .." w79 {
      tunnel: w100 -> [w135 _]
      tunnel: w87 -> [w132 _]
      tunnel: [w131 i32[] [0, 0, 0, 0, 0, 0, 0, 0, 0, 0, 0, 0] ("value")] -> w77
      frame No Error {
        n65 = Index Array(array=w135, index=0) -> (element=w133:string)
        n66 = Unflatten From XML(xml string=w133, type=w132) -> (value=w131:i32[])  [unwired: 1 in, 1 out]
      }
      frame Error {
      }
    }
    n67 = First Call?() -> (First Call?: T/F=w119:bool)
    n68 = Select(t=w77, s=w119, f=w93) -> (s? t:f=w76:i32[])
    n69 = Add(x=w76, y=w75) -> (x+y=w78:i32[])
    n70 = Index Array(array=w78, index #1=0 ("index")) -> (element #1=w84:i32, element #2=w83:i32, element #3=w82:i32, element #4=w81:i32, element #5=w72:i32, element #6=w71:i32, element #7=w70:i32, element #8=w69:i32, element #9=w66:i32, element #10=w65:i32, element #11=w64:i32, element #12=w63:i32)  [unwired: 11 in]
    n71 = Unbundle(w80) -> ("Ret_Power_Port_Left"=w85:refnum<vi>, "Ret_Power_Port_Right"=w86:refnum<vi>, "Ret_Ball_Left"=w68:refnum<vi>, "Ret_Ball_Right"=w67:refnum<vi>, "Ret_Feeder_Left"=w60:refnum<vi>, "Ret_Feeder_Right"=w59:refnum<vi>)
    n72 = Flatten To XML(6:w76) -> (2:w106:string)
    n73 = call "EdgeTrigger.vi"("Input Signal"="Save") -> ("Rising Edge Trigger"=w57:bool)  [unwired: 2 out]
    n74 = case shown="True" w57 {
      tunnel: w106 -> [_ w138]
      tunnel: w101 -> [_ w137]
      frame False {
      }
      frame True {
        n75 = call-poly <vilib>:"Write to XML File.vi"("XML Input"=w138, "XML File Path"=w137) -> ()  [unwired: 7 in, 3 out]
      }
    }
    n76 = property class="Bool (strict)"(reference=w85, "Left"=w84, "Top"=w83) -> ()  [unwired: 1 in, 2 out]
    n77 = property class="Bool (strict)"(reference=w86, "Left"=w82, "Top"=w81) -> ()  [unwired: 1 in, 2 out]
    n78 = property class="Bool (strict)"(reference=w68, "Left"=w72, "Top"=w71) -> ()  [unwired: 1 in, 2 out]
    n79 = property class="Bool (strict)"(reference=w67, "Left"=w70, "Top"=w69) -> ()  [unwired: 1 in, 2 out]
    n80 = property class="Bool (strict)"(reference=w60, "Left"=w66, "Top"=w65) -> ()  [unwired: 1 in, 2 out]
    n81 = property class="Bool (strict)"(reference=w59, "Left"=w64, "Top"=w63) -> ()  [unwired: 1 in, 2 out]
  }
  n82 = while {
    tunnel: w9 -> [w201]
    tunnel: w6 -> [w182]
    tunnel: w2 -> [w179]
    stop <- FALSE stop-if-true
    w160 = "320x240 MJPEG 22 fps" ("String")
    w159 = "mjpg:http://10.42.65.93:5800"
    w162 = "/CameraPublisher/limelight/"
    # "manually configure the NT for a single LimeLight\ncamera in order to bypass WPILib's camera\nauto-detection which fails when the NTs are refreshed\nafter the code restarts on the roboRIO"
    # "Camera Feeds"
    n83 = Concatenate Strings("ip:http://", "10.42.65.93:5800" ("string")) -> (w173:string)
    n84 = Build Array(w159, w159) -> (w171:string[])
    n85 = local read "NT Connection"() -> (w178:bool)
    n86 = local read "Rec Mode"() -> (w202:enum32{"Stop", "Record", "Playback"})
    n87 = Concatenate Strings(w162, "source") -> (w174:string)
    n88 = Concatenate Strings(w162, "description") -> (w169:string)
    n89 = Concatenate Strings(w162, "mode") -> (w166:string)
    n90 = Build Array(w160) -> (w161:string[])
    n91 = Concatenate Strings(w162, "streams") -> (w172:string)
    n92 = Concatenate Strings(w162, "modes") -> (w164:string)
    n93 = Bundle("Camera Name"="Camera Name", w182, "Saved DB Images Info"=w201) -> (w200:T14)  [unwired: 1 in]
    n94 = call-poly <vilib>:"NT Write Value.vi"("String"=w173, "Name"=w174) -> ()  [unwired: 9 in, 1 out]
    n95 = call-poly <vilib>:"NT Write Value.vi"("String"="limelight", "Name"=w169) -> ()  [unwired: 9 in, 1 out]
    n96 = call-poly <vilib>:"NT Write Value.vi"("String"=w160, "Name"=w166) -> ()  [unwired: 9 in, 1 out]
    n97 = call-poly <vilib>:"NT Write Value.vi"("String Array"=w171, "Name"=w172) -> ()  [unwired: 9 in, 1 out]
    n98 = call-poly <vilib>:"NT Write Value.vi"("String Array"=w161, "Name"=w164) -> ()  [unwired: 9 in, 1 out]
    n99 = control-ref of="Camera Perf"() -> (w198:refnum<vi>)
    n100 = call <vilib>:"WPI_CameraRead MJPG for Dashboard_2.vi"("Camera Settings"="Camera Settings", "Rec Mode"=w202, "NT Connection"=w178, "Capture Info"=w200, "Image in"=w179) -> ("perf info"=w199:cluster{"Bandwidth (Mbps)":dbl, "fps":dbl}, "Active"=w181:bool, "Image\\ out"=w203:T3)  [unwired: 4 in]
    n101 = call <vilib>:"WPI_DashboardFormatPerf.vi"("Right Camera Perf"=cluster{"Bandwidth (Mbps)":dbl, "FPS":dbl} {"Bandwidth (Mbps)"=0.0, "FPS"=0.0}, "Performance"=w199, "String in"=w198) -> ()  [unwired: 9 in]
    n102 = case shown="True" w181 {
      tunnel: w203 -> [w216 w219]
      tunnel: [w216 w218] -> w197
      frame False {
        n103 = Wait Until Next ms Multiple(millisecond multiple=u32 500) -> ()  [unwired: 1 out]
      }
      frame True {
        # "image annotation etc."
        n104 = call "IMAQ Clear Overlay"("Image"=w219) -> ("Image Out"=w218:T3)  [unwired: 2 in, 8 out]
      }
    }
    n105 = Not(x=w181) -> (.not. x?=→"Camera_1_Fault":bool)
    n106 = call "IMAQ Rotate"("Angle (degrees)"=sgl 0.0, "Image Src"=w197) -> ("Image Dst Out"=w187:T3)  [unwired: 8 in, 1 out]
    n107 = call "IMAQ GetImageSize"("Image"=w187) -> ("Y Resolution"=w183:i32, "X Resolution"=w193:i32)  [unwired: 3 in, 1 out]
    n108 = To Double Precision Float(number=w193) -> (double precision float=w195:dbl)
    n109 = To Double Precision Float(number=w183) -> (double precision float=w194:dbl)
    n110 = Divide(x=w195, y=w194) -> (x/y=w192:dbl)
    n111 = Less?(x=w192, y=1.5) -> (x < y?=w184:bool)
    "Camera_2_Fault" <- w184
    n112 = case shown="False" w184 {
      tunnel: "Partial Video Stream" ("Image Name") -> [_ w215]
      tunnel: [w205 w214] -> w186
      tunnel: w187 -> [w205 w210]
      frame False {
        # "wide angle camera found"
      }
      frame True {
        # "no wide angle camera found"
        n113 = call "IMAQ GetImageInfo"("Image"=w210) -> ("Y Resolution"=w209:i32, "X Resolution"=w208:i32, "Image Type"=w213:T12)  [unwired: 3 in, 5 out]
        n114 = call "IMAQ Create"("Image Name"=w215, "Image Type"=w213) -> ("New Image"=w212:T3)  [unwired: 3 in, 1 out]
        n115 = Multiply(x=w208, y=2) -> (x*y=w207:i32)
        n116 = call "IMAQ SetImageSize"("Y Resolution"=w209, "X Resolution"=w207, "Image"=w212) -> ("Image Out"=w211:T3)  [unwired: 2 in, 1 out]
        n117 = call "IMAQ ImageToImage 2"("Image Src (Small)"=w210, "Image Src (Large)"=w211) -> ("Image Dst Out"=w214:T3)  [unwired: 8 in, 1 out]
      }
    }
    "Combined Camera Feed" <- w186
  }
  n118 = while {
    tunnel: w8 -> [w223]
    tunnel: w22 -> [w220]
    stop <- FALSE stop-if-true
    # "Primary Indicators and Controls"
    n119 = call <vilib>:"WPI_DashboardRetrieveStatusInfo.vi"("Binding Refnum"=w223, "Window Mode Notifier"=w220, "TCP Cnx"="TCP") -> ("Power and Errors"=w224:T17, "Robot Metrics"=w227:T18, "Status Info"=w228:T19, "Control Info"=w225:T20, "Robot Mode"=w222:T7, "Process?"=w226:bool)  [unwired: 3 in]
    "Mode" <- w222
    n120 = case shown="True" w226 {
      tunnel: w228 -> [_ _]
      tunnel: w227 -> [_ _]
      tunnel: w225 -> [_ _]
      tunnel: w224 -> [_ _]
      tunnel: w222 -> [_ _]
      frame False {
        n121 = Wait (ms)(milliseconds to wait=u32 20) -> ()  [unwired: 1 out]
      }
      frame True {
        n122 = stacked-sequence {
          frame #0 {
            # "general reporting"
            # "resource utilization"
            # "autonomous reporting"
            # "report match time"
            # "report robot status and resource utilization"
            n123 = call-poly <vilib>:"NT Read Value.vi"("Name"="Battery_Critical") -> ("Boolean"=→"Battery_Critical":bool)  [unwired: 9 in, 1 out]
            n124 = call-poly <vilib>:"NT Read Value.vi"("Name"="Diverting_Power") -> ("Boolean"=→"Diverting_Power":bool)  [unwired: 9 in, 1 out]
            n125 = call-poly <vilib>:"NT Read Value.vi"("Name"="Electrical_Fault") -> ("Boolean"=→"Electrical_Fault":bool)  [unwired: 9 in, 1 out]
            n126 = call-poly <vilib>:"NT Read Value.vi"("Name"="CAN_Bus_Fault") -> ("Boolean"=→"CAN_Bus_Fault":bool)  [unwired: 9 in, 1 out]
            n127 = call-poly <vilib>:"NT Read Value.vi"("Name"="Control_Latency_Alarm") -> ("Boolean"=w293:bool)  [unwired: 9 in, 1 out]
            "Slow_Loop" <- w293
            n128 = call-poly <vilib>:"NT Read Value.vi"("Name"="Control_Loop_Time") -> ("Numeric"=w283:dbl)  [unwired: 9 in, 1 out]
            n129 = call-poly <vilib>:"NT Read Value.vi"("Name"="Pose_Loop_Time") -> ("Numeric"=w294:dbl)  [unwired: 9 in, 1 out]
            n130 = call-poly <vilib>:"NT Read Value.vi"("Name"="Compressor_On") -> ("Boolean"=→"Compressor_On":bool)  [unwired: 9 in, 1 out]
            n131 = call-poly <vilib>:"NT Read Value.vi"("Name"="Pressure_Vent") -> ("Boolean"=→"Pressure_Vent":bool)  [unwired: 9 in, 1 out]
            n132 = call-poly <vilib>:"NT Read Value.vi"("Name"="Pressure_Transducer") -> ("Numeric"=→"Pressure_Transducer":dbl)  [unwired: 9 in, 1 out]
            n133 = call-poly <vilib>:"NT Read Value.vi"("Default Value"=13.0, "Name"="Battery_Voltage") -> ("Numeric"=→"Battery_Voltage":dbl)  [unwired: 8 in, 1 out]
            n134 = call-poly <vilib>:"NT Read Value.vi"("Name"="Pressure_Leak") -> ("Boolean"=→"Pressure_Leak":bool)  [unwired: 9 in, 1 out]
            n135 = To Unsigned Long Integer(number=w294) -> (unsigned 32bit integer=→"Pose Loop Time (ms)":u32)
            n136 = To Unsigned Long Integer(number=w283) -> (unsigned 32bit integer=→"Control Loop Time (ms)":u32)
            n137 = Select(t=u32 16711680 ("Numeric Text.Text Colors:Text Color"), s=w293, f=u32 4934475 ("Numeric Text.Text Colors:Text Color")) -> (s? t:f=w288:u32)
            n138 = property on="Control Loop Time (ms)" class="DigNum (strict)"("NumText.BG Color"=w288) -> ()  [unwired: 2 in, 2 out]
            n139 = call-poly <vilib>:"NT Read Value.vi"("Name"="Auto_Error") -> ("Boolean"=→"Auto_Error":bool)  [unwired: 9 in, 1 out]
            n140 = call-poly <vilib>:"NT Read Value.vi"("Name"="Robot_is_Autonomous") -> ("Boolean"=→"Robot_is_Autonomous_0" →"Robot_is_Autonomous_1" →"Robot_is_Autonomous_2":bool)  [unwired: 9 in, 1 out]
            n141 = call-poly <vilib>:"NT Read Value.vi"("Name"="Auto_Manipulator_Action") -> ("String"=→"Manipulator Action":string)  [unwired: 9 in, 1 out]
            n142 = call-poly <vilib>:"NT Read Value.vi"("Name"="Auto_Drive_Action") -> ("String"=→"Drive Action":string)  [unwired: 9 in, 1 out]
            n143 = call-poly <vilib>:"NT Read Value.vi"("Default Value"=0.0, "Name"="Remaining_Time") -> ("Numeric"=w267:dbl)  [unwired: 8 in, 1 out]
            n144 = call-poly <vilib>:"NT Read Value.vi"("Name"="Robot_Mode") -> ("String"=w265:string)  [unwired: 9 in, 1 out]
            n145 = Equal?(x=w265, y="Teleop Enabled") -> (x = y?=w266:bool)
            n146 = Greater Or Equal To 0?(x=w267) -> (x >= 0?=w268:bool)
            n147 = Less?(x=w267, y="Warning Time (s)") -> (x < y?=w259:bool)
            n148 = Compound Arithmetic op=AND(w268, w259, w266) -> (w264:bool)
            "Match_End" <- w264
            n149 = call "BlinkLight.vi"() -> ("Blinked"=w258:bool)  [unwired: 1 in]
            n150 = In Range and Coerce(upper limit=inf, x=w267, lower limit=0.0) -> (coerced(x)=w260:dbl)  [unwired: 1 out]
            n151 = To Single Precision Float(number=w260) -> (single precision float=→"Match Time(s)":sgl)
            n152 = Select(t=w258, s=w264, f=FALSE) -> (s? t:f=w263:bool)
            n153 = Select(t=u32 16760064 ("Numeric Text.Text Colors:Text Color"), s=w263, f=u32 16448250 ("Numeric Text.Text Colors:Text Color")) -> (s? t:f=w262:u32)
            n154 = property on="Match Time(s)" class="DigNum (strict)"("NumText.TextColor"=w262) -> ()  [unwired: 2 in, 2 out]
            n155 = local read "Dashboard Tab"() -> (w235:T1)
            n156 = Equal?(x=w235, y=T1."Tune") -> (x = y?=w236:bool)
            n157 = call-poly <vilib>:"NT Read Value.vi"("Default Value"="No robot code versioning information...", "Name"="Robot_Code_Version") -> ("String"=→"Robot_Code_Version":string)  [unwired: 8 in, 1 out]
            n158 = call-poly <vilib>:"NT Write Value.vi"("Boolean"=w236, "Name"="Tune_Tab") -> ()  [unwired: 9 in, 1 out]
          }
          frame #1 {
            # "targeting data"
            # "report robot pose and targeting data"
            n159 = call-poly <vilib>:"NT Read Value.vi"("Name"="Alliance_Color") -> ("Numeric"=w310:dbl)  [unwired: 9 in, 1 out]
            n160 = To Unsigned Word Integer(number=w310) -> (unsigned 16bit integer=w311:u16)
            n161 = call-poly <vilib>:"NT Read Value.vi"("Default Value"=-1.0, "Name"="Robot_Y") -> ("Numeric"=w334:dbl)  [unwired: 8 in, 1 out]
            "Robot Y" <- w334
            n162 = call-poly <vilib>:"NT Read Value.vi"("Default Value"=-1.0, "Name"="Robot_X") -> ("Numeric"=w333:dbl)  [unwired: 8 in, 1 out]
            "Robot X" <- w333
            n163 = call-poly <vilib>:"NT Read Value.vi"("Default Value"=0.0, "Name"="Robot_H") -> ("Numeric"=w335:dbl)  [unwired: 8 in, 1 out]
            n164 = feedback #1(w311) -> (w306:u16)
            n165 = feedback-in #1(w311) -> ()
            n166 = Not Equal?(x=w311, y=w306) -> (x != y?=w308:bool)
            n167 = feedback #2("Field Map") -> (w312:u16)
            n168 = feedback-in #2("Field Map") -> ()
            n169 = Not Equal?(x="Field Map", y=w312) -> (x != y?=w314:bool)
            n170 = call-poly <vilib>:"NT Read Value.vi"("Name"="Robot_Mode") -> ("String"=w336:string)  [unwired: 9 in, 1 out]
            n171 = Quotient & Remainder(x=w335, y=360.0) -> (x-y*floor(x/y)=→"Robot H":dbl)  [unwired: 1 out]
            n172 = First Call?() -> (First Call?: T/F=w307:bool)
            n173 = call "EdgeTrigger.vi"("Input Signal"="Export_Robot_Pose") -> ("Rising Edge Trigger"=w315:bool)  [unwired: 2 out]
            n174 = Compound Arithmetic op=OR(w308, w307, w314) -> (w309:bool)
            n175 = case shown="True" w309 {
              tunnel: w311 -> [_ w349]
              tunnel: "Field Map" -> [_ w347]
              frame False {
              }
              frame True {
                # "load and display a field map"
                n176 = To Long Integer(number=w347) -> (32bit integer=w345:i32)
                n177 = Current VI's Path() -> (path=w352:path)
                n178 = Strip Path(path=w352) -> (stripped path=w351:path)  [unwired: 1 out]
                n179 = Strip Path(path=w351) -> (stripped path=w348:path)  [unwired: 1 out]
                n180 = List Folder(path=w348, pattern="*map*.png") -> (filenames=w346:string[])  [unwired: 2 in, 3 out]
                n181 = Index Array(array=w346, index=w345) -> (element=w344:string)
                n182 = property on="Field Map" class="Ring (strict)"("Strings []"=w346) -> ()  [unwired: 2 in, 2 out]
                n183 = Build Path(base path=w348, name or relative path=w344) -> (appended path=w350:path)
                n184 = call <vilib>:"Read PNG File.vi"("path to PNG file"=w350) -> ("error out"=w354:errorcluster, "image data"=w353:T21)  [unwired: 8 in, 1 out]
                n185 = case shown="No Error" w354 {
                  tunnel: w353 -> [w372 _]
                  tunnel: w349 -> [w356 _]
                  frame No Error {
                    w373 = T12 4 items=["Grayscale (U8)", "Grayscale (I16)", "Grayscale (SGL)", "Complex (CSG)", "RGB (U32)", "HSL (U32)", "RGB (U64)", "Grayscale (U16)"] ("Image Type")
                    n186 = call <vilib>:"Unflatten Pixmap.vi"("image data"=w372) -> ("24-bit pixmap"=w371:u32[][])  [unwired: 4 in, 6 out]
                    n187 = property on="Robot Pose" class="XYGraph (strict)"() -> ("Width"=w376:u32, "Height"=w375:u32)  [unwired: 2 in, 2 out]
                    n188 = call "IMAQ Create"("Image Name"="field", "Image Type"=w373) -> ("New Image"=w370:T3)  [unwired: 3 in, 1 out]
                    n189 = Equal?(x=w356, y=WPI_DriverStationAllianceInfo."Red" ("x")) -> (x = y?=w358:bool)
                    n190 = call "IMAQ ArrayToColorImage"("Image Pixels (U32)"=w371, "Image"=w370) -> ("Image Out"=w369:T3)  [unwired: 3 in, 1 out]
                    n191 = To Long Integer(number=w376) -> (32bit integer=w365:i32)
                    n192 = To Long Integer(number=w375) -> (32bit integer=w366:i32)
                    n193 = call "IMAQ Resample"("X Resolution"=w365, "Y Resolution"=w366, "Image Src"=w369) -> ("Image Dst Out"=w364:T3)  [unwired: 7 in, 1 out]
                    n194 = Select(t=180.0, s=w358, f=0.0) -> (s? t:f=w362:dbl)
                    n195 = To Single Precision Float(number=w362) -> (single precision float=w361:sgl)
                    n196 = call "IMAQ Rotate"("Angle (degrees)"=w361, "Image Src"=w364) -> ("Image Dst Out"=w363:T3)  [unwired: 8 in, 1 out]
                    n197 = call "IMAQ ColorImageToArray"("Image"=w363) -> ("Image Pixels (U32)"=w368:u32[][])  [unwired: 3 in, 2 out]
                    n198 = call <vilib>:"Flatten Pixmap.vi"("24-bit pixmap"=w368) -> ("image data"=w367:T21)  [unwired: 10 in]
                    n199 = call <vilib>:"Draw Flattened Pixmap.vi"("image data"=w367) -> ("new picture"=w355:picture)  [unwired: 8 in]
                    n200 = property on="Robot Pose" class="XYGraph (strict)"("PlotImages.Back"=w355) -> ()  [unwired: 2 in, 2 out]
                    n201 = property on="Robot Pose 1" class="XYGraph (strict)"("PlotImages.Back"=w355) -> ()  [unwired: 2 in, 2 out]
                  }
                  frame Error {
                  }
                }
              }
            }
            n202 = case shown="True" w315 {
              frame False {
              }
              frame True {
                # "export the current robot pose data"
                n203 = Get Date/Time In Seconds() -> (seconds since 1Jan1904=w390:timestamp)
                n204 = Format Date/Time String(time format string (%c)="%Y-%m-%d_%H-%M", seconds (now)=w390) -> (date/time string=w388:string)  [unwired: 1 in]
                n205 = Concatenate Strings("robot pose data " ("string"), w388) -> (w386:string)
                n206 = Current VI's Path() -> (path=w385:path)
                n207 = String To Path(string=w386) -> (path=w382:path)
                n208 = Strip Path(path=w385) -> (stripped path=w384:path)  [unwired: 1 out]
                n209 = Strip Path(path=w384) -> (stripped path=w383:path)  [unwired: 1 out]
                n210 = Build Path(base path=w383, name or relative path=w382) -> (appended path=w381:path)
                n211 = invoke on="Robot Pose" class="XYGraph (strict)" method="Export Image"("FileType"=enum32{"BMP", "EPS", "EMF", "PICT"}."BMP" ("File Type"), "Target"=enum32{"File", "Clipboard"}."File", "Path"=w381, "HideGrid"=TRUE ("Hide Grid"), "Overwrite"=TRUE ("Always Overwrite")) -> ()  [unwired: 3 in, 8 out]
              }
            }
            n212 = Equal?(x=w336, y="Teleop Enabled") -> (x = y?=w337:bool)
            n213 = Equal?(x=w336, y="Autonomous Enabled") -> (x = y?=w339:bool)
            n214 = Or(x=w339, y=w337) -> (x .or. y?=w338:bool)
            n215 = call "EdgeTrigger.vi"("Input Signal"=w339) -> ("Rising Edge Trigger"=w341:bool)  [unwired: 2 out]
            n216 = Or(x="Clear_Robot_Pose_Display", y=w341) -> (x .or. y?=w342:bool)
            n217 = call "RenderRobotPose.vi"("Robot X (in)"=w333, "Robot Width (in)"=30.5 ("Robot Size (in)"), "Robot Length (in)"=30.5 ("Robot Width (in)"), "Buffer Time (min)"=5.0, "Robot Y (in)"=w334, "Robot Heading (deg)"=w335, "Turret Heading (deg)"=0.0, "Robot Enabled"=w338, "Reset"=w342) -> ("Robot Pose"=→"Robot Pose" →"Robot Pose 1":cluster{dbl[], dbl[]}[])  [unwired: 6 in]
            n218 = call-poly <vilib>:"NT Read Value.vi"("Name"="LL_Valid") -> ("Boolean"=→"LL_Valid":bool)  [unwired: 9 in, 1 out]
            n219 = call-poly <vilib>:"NT Read Value.vi"("Name"="Distance_To_Target") -> ("Numeric"=→"Distance_To_Target_Detail":dbl)  [unwired: 9 in, 1 out]
            n220 = local read "Robot_is_Autonomous_0"() -> (w299:bool)
            n221 = Not(x="Hide_Popups") -> (.not. x?=w300:bool)
            n222 = And(x=w300, y=w299) -> (x .and. y?=w298:bool)
            n223 = property on="Robot Pose 1" class="XYGraph (strict)"("Visible"=w298) -> ()  [unwired: 2 in, 2 out]
          }
          frame #2 {
            # "driver control configuration"
            # "robot configuration"
            # "robot and driver control configuration"
            n224 = Build Array("N/A") -> (w419:string[])
            n225 = Build Array("N/A") -> (w415:string[])
            n226 = To Double Precision Float(number="Robot Profile") -> (double precision float=w412:dbl)
            n227 = call-poly <vilib>:"NT Read Value.vi"("Default Value"=w419, "Name"="Legal_Pipelines") -> ("String Array"=w418:string[])  [unwired: 8 in, 1 out]
            n228 = call-poly <vilib>:"NT Read Value.vi"("Default Value"=w415, "Name"="Legal_Robots") -> ("String Array"=w414:string[])  [unwired: 8 in, 1 out]
            n229 = call-poly <vilib>:"NT Write Value.vi"("Numeric"=w412, "Name"="Selected_Robot") -> ()  [unwired: 9 in, 1 out]
            n230 = To Double Precision Float(number="Default Camera Pipeline") -> (double precision float=w416:dbl)
            n231 = property on="Default Camera Pipeline" class="Ring (strict)"("Strings []"=w418) -> ()  [unwired: 2 in, 2 out]
            n232 = property on="Robot Profile" class="Ring (strict)"("Strings []"=w414) -> ()  [unwired: 2 in, 2 out]
            n233 = call-poly <vilib>:"NT Write Value.vi"("Numeric"=w416, "Name"="Selected_Default_Pipeline") -> ()  [unwired: 9 in, 1 out]
            n234 = Build Array("N/A") -> (w400:string[])
            n235 = And(x="Calibrate_Joysticks", y="Arm_Calibrate_Joysticks") -> (x .and. y?=w404:bool)
            n236 = To Double Precision Float(number="Driver Profile") -> (double precision float=w397:dbl)
            n237 = call-poly <vilib>:"NT Read Value.vi"("Default Value"=w400, "Name"="Legal_Drivers") -> ("String Array"=w399:string[])  [unwired: 8 in, 1 out]
            "Legal_Drivers" <- w399
            n238 = Not(x="Arm_Calibrate_Joysticks") -> (.not. x?=w402:bool)
            n239 = call-poly <vilib>:"NT Write Value.vi"("Numeric"=w397, "Name"="Selected_Driver") -> ()  [unwired: 9 in, 1 out]
            n240 = property on="Driver Profile" class="Ring (strict)"("Strings []"=w399) -> ()  [unwired: 2 in, 2 out]
            n241 = call-poly <vilib>:"NT Write Value.vi"("Boolean"=w404, "Name"="Calibrate_Joysticks") -> ()  [unwired: 9 in, 1 out]
            n242 = Select(t=cluster{u32, u32}[] [{11776947, 16448250}, {16448250, 16448250}] ("Colors [4]"), s=w402, f=cluster{u32, u32}[] [{6618880, 16448250}, {16448250, 16448250}] ("Colors [4]")) -> (s? t:f=w403:cluster{u32, u32}[])
            n243 = property on="Calibrate_Joysticks" class="Bool"("Colors [4]"=w403) -> ()  [unwired: 2 in, 2 out]
          }
          frame #3 {
            # "configure auto play"
            # "set robot pose"
            # "autonomous configuration"
            n244 = call-poly <vilib>:"NT Write Value.vi"("Numeric"="Manual_Start_X", "Name"="Manual_Start_X") -> ()  [unwired: 9 in, 1 out]
            n245 = call-poly <vilib>:"NT Write Value.vi"("Numeric"="Manual_Start_Y", "Name"="Manual_Start_Y") -> ()  [unwired: 9 in, 1 out]
            n246 = call-poly <vilib>:"NT Write Value.vi"("Numeric"="Manual_Start_H", "Name"="Manual_Start_H") -> ()  [unwired: 9 in, 1 out]
            n247 = call-poly <vilib>:"NT Write Value.vi"("Boolean"="Disable_Fusion_X", "Name"="Disable_Fusion_X") -> ()  [unwired: 9 in, 1 out]
            n248 = call-poly <vilib>:"NT Write Value.vi"("Boolean"="Disable_Fusion_Y", "Name"="Disable_Fusion_Y") -> ()  [unwired: 9 in, 1 out]
            n249 = call-poly <vilib>:"NT Write Value.vi"("Boolean"="Push_Robot_Start", "Name"="Push_Robot_Start") -> ()  [unwired: 9 in, 1 out]
            n250 = To Double Precision Float(number="Autonomous Play") -> (double precision float=w428:dbl)
            n251 = Build Array("N/A") -> (w430:string[])
            n252 = call-poly <vilib>:"NT Read Value.vi"("Default Value"="Waiting for connection...", "Name"="Auto_Playbook") -> ("String"=→"Auto Playbook Entry":string)  [unwired: 8 in, 1 out]
            n253 = call-poly <vilib>:"NT Read Value.vi"("Name"="Auto_Path_Suffix") -> ("String"=→"Auto_Suffix":string)  [unwired: 9 in, 1 out]
            n254 = call-poly <vilib>:"NT Read Value.vi"("Default Value"=w430, "Name"="Legal_Auto_Plays") -> ("String Array"=w431:string[])  [unwired: 8 in, 1 out]
            n255 = call-poly <vilib>:"NT Write Value.vi"("Numeric"="Auto_Delay", "Name"="Auto_Delay") -> ()  [unwired: 9 in, 1 out]
            n256 = call-poly <vilib>:"NT Write Value.vi"("Numeric"=w428, "Name"="Selected_Auto_Play") -> ()  [unwired: 9 in, 1 out]
            n257 = call-poly <vilib>:"NT Write Value.vi"("Boolean"="Auto_Test_Mode", "Name"="Auto_Test_Mode") -> ()  [unwired: 9 in, 1 out]
            n258 = call-poly <vilib>:"NT Write Value.vi"("Boolean"="Force_Human_Control", "Name"="Force_Human_Control") -> ()  [unwired: 9 in, 1 out]
            n259 = call-poly <vilib>:"NT Write Value.vi"("Boolean"="Refresh_Auto_Play_List", "Name"="Refresh_Auto_Play_List") -> ()  [unwired: 9 in, 1 out]
            n260 = property on="Autonomous Play" class="Ring (strict)"("Strings []"=w431) -> ()  [unwired: 2 in, 2 out]
          }
          frame #4 {
            w457 = cluster{u32, u32}[] [{15663313, 16448250}, {16448250, 16448250}] ("Un-selected Color")
            w491 = cluster{u32, u32}[] [{9567230, 16448250}, {16448250, 16448250}] ("Un-selected Color")
            # "shooter state controller"
            # "ball handling and shooter controls"
            # "master state controller"
            # "manipulator commands"
            n261 = local read "Arm_Climber"() -> (w506:bool)
            n262 = call-poly <vilib>:"NT Read Value.vi"("Name"="Confirmed_States") -> ("Boolean Array"=w495:bool[])  [unwired: 9 in, 1 out]
            n263 = call-poly <vilib>:"NT Read Value.vi"("Name"="Disallowed_States") -> ("Boolean Array"=w496:bool[])  [unwired: 9 in, 1 out]
            n264 = And(x="State_Climb", y="Arm_Climber") -> (x .and. y?=w509:bool)
            n265 = Index Array(array=w496, index #1=0 ("index")) -> (element #1=w498:bool, element #2=w501:bool, element #3=w514:bool, element #4=w510:bool)  [unwired: 3 in]
            n266 = Index Array(array=w495, index #1=0 ("index")) -> (element #1=w497:bool, element #2=w500:bool, element #3=w513:bool, element #4=w511:bool)  [unwired: 3 in]
            n267 = Not(x=w506) -> (.not. x?=w507:bool)
            n268 = Build Array("State_Normal", "State_Rotation_Control", "State_Position_Control", w509) -> (w494:bool[])
            n269 = Or(x=w510, y=w507) -> (x .or. y?=w505:bool)
            n270 = call "ButtonColorChooser.vi"("Un-selected Color"=w491, "Disallowed"=w498, "Confirmed"=w497) -> ("Final Color"=w499:cluster{u32, u32}[])  [unwired: 8 in]
            n271 = call "ButtonColorChooser.vi"("Un-selected Color"=w491, "Disallowed"=w501, "Confirmed"=w500) -> ("Final Color"=w503:cluster{u32, u32}[])  [unwired: 8 in]
            n272 = call "ButtonColorChooser.vi"("Un-selected Color"=w491, "Disallowed"=w505, "Confirmed"=w511) -> ("Final Color"=w502:cluster{u32, u32}[])  [unwired: 8 in]
            n273 = call "ButtonColorChooser.vi"("Un-selected Color"=w491, "Disallowed"=w514, "Confirmed"=w513) -> ("Final Color"=w512:cluster{u32, u32}[])  [unwired: 8 in]
            n274 = call-poly <vilib>:"NT Write Value.vi"("Boolean Array"=w494, "Name"="DS_States") -> ()  [unwired: 9 in, 1 out]
            n275 = property on="State_Normal" class="Bool"("Colors [4]"=w499) -> ()  [unwired: 2 in, 2 out]
            n276 = property on="State_Climb" class="Bool"("Colors [4]"=w502) -> ()  [unwired: 2 in, 2 out]
            n277 = property on="State_Rotation_Control" class="Bool"("Colors [4]"=w503) -> ()  [unwired: 2 in, 2 out]
            n278 = property on="State_Position_Control" class="Bool"("Colors [4]"=w512) -> ()  [unwired: 2 in, 2 out]
            n279 = call-poly <vilib>:"NT Write Value.vi"("Boolean"="Pre_Spin", "Name"="Pre_Spin") -> ()  [unwired: 9 in, 1 out]
            n280 = call-poly <vilib>:"NT Write Value.vi"("Boolean"="Clear_Jams", "Name"="Clear_Jams") -> ()  [unwired: 9 in, 1 out]
            n281 = call-poly <vilib>:"NT Read Value.vi"("Name"="Confirmed_Shooter_States") -> ("Boolean Array"=w464:bool[])  [unwired: 9 in, 1 out]
            n282 = call-poly <vilib>:"NT Read Value.vi"("Name"="Disallowed_Shooter_States") -> ("Boolean Array"=w465:bool[])  [unwired: 9 in, 1 out]
            n283 = Build Array("Mode_TargetingComputer", "Mode_Wall", "Mode_InitiationLine", "Mode_CloseTrench", "Mode_FarTrench") -> (w458:bool[])
            n284 = Index Array(array=w465, index #1=0 ("index")) -> (element #1=w467:bool, element #2=w470:bool, element #3=w474:bool, element #4=w479:bool, element #5=w480:bool)  [unwired: 4 in]
            n285 = Index Array(array=w464, index #1=0 ("index")) -> (element #1=w466:bool, element #2=w469:bool, element #3=w471:bool, element #4=w477:bool, element #5=w478:bool)  [unwired: 4 in]
            n286 = call-poly <vilib>:"NT Write Value.vi"("Boolean Array"=w458, "Name"="DS_Shooter_States") -> ()  [unwired: 9 in, 1 out]
            n287 = call "ButtonColorChooser.vi"("Un-selected Color"=w457, "Disallowed"=w467, "Confirmed"=w466) -> ("Final Color"=w468:cluster{u32, u32}[])  [unwired: 8 in]
            n288 = call "ButtonColorChooser.vi"("Un-selected Color"=w457, "Disallowed"=w470, "Confirmed"=w469) -> ("Final Color"=w473:cluster{u32, u32}[])  [unwired: 8 in]
            n289 = call "ButtonColorChooser.vi"("Un-selected Color"=w457, "Disallowed"=w474, "Confirmed"=w471) -> ("Final Color"=w472:cluster{u32, u32}[])  [unwired: 8 in]
            n290 = call "ButtonColorChooser.vi"("Un-selected Color"=w457, "Disallowed"=w479, "Confirmed"=w477) -> ("Final Color"=w475:cluster{u32, u32}[])  [unwired: 8 in]
            n291 = call "ButtonColorChooser.vi"("Un-selected Color"=w457, "Disallowed"=w480, "Confirmed"=w478) -> ("Final Color"=w476:cluster{u32, u32}[])  [unwired: 8 in]
            n292 = property on="Mode_TargetingComputer" class="Bool"("Colors [4]"=w468) -> ()  [unwired: 2 in, 2 out]
            n293 = property on="Mode_InitiationLine" class="Bool"("Colors [4]"=w472) -> ()  [unwired: 2 in, 2 out]
            n294 = property on="Mode_CloseTrench" class="Bool"("Colors [4]"=w475) -> ()  [unwired: 2 in, 2 out]
            n295 = property on="Mode_FarTrench" class="Bool"("Colors [4]"=w476) -> ()  [unwired: 2 in, 2 out]
            n296 = property on="Mode_Wall" class="Bool"("Colors [4]"=w473) -> ()  [unwired: 2 in, 2 out]
          }
          frame #5 {
            # "actuator test interlocks"
            # "emergency overrides"
            # "emergency overrides and interlocks"
            n297 = And(x="Master_Safety_Override_1", y="Master_Safety_Override_2") -> (x .and. y?=w538:bool)
            n298 = call-poly <vilib>:"NT Read Value.vi"("Name"="Tablet_Override") -> ("Boolean"=→"Tablet_Override":bool)  [unwired: 9 in, 1 out]
            n299 = call-poly <vilib>:"NT Write Value.vi"("Boolean"="Clear_Errors", "Name"="Clear_Errors") -> ()  [unwired: 9 in, 1 out]
            n300 = call-poly <vilib>:"NT Write Value.vi"("Boolean"="Super_Test_Mode", "Name"="Super_Test_Mode") -> ()  [unwired: 9 in, 1 out]
            n301 = call-poly <vilib>:"NT Write Value.vi"("Boolean"="Camera_Override", "Name"="Camera_Override") -> ()  [unwired: 9 in, 1 out]
            n302 = call-poly <vilib>:"NT Write Value.vi"("Boolean"="Auto_Target_Override", "Name"="Auto_Target_Override") -> ()  [unwired: 9 in, 1 out]
            n303 = call-poly <vilib>:"NT Write Value.vi"("Boolean"="Field_Oriented_Override", "Name"="Field_Oriented_Override") -> ()  [unwired: 9 in, 1 out]
            n304 = call-poly <vilib>:"NT Write Value.vi"("Boolean"=w538, "Name"="Master_Safety_Override") -> ()  [unwired: 9 in, 1 out]
            n305 = property on="Actuator Testing" class="Ring (strict)"() -> ("RingText.Text"=w527:string)  [unwired: 2 in, 2 out]
            n306 = Build Array("No_Test") -> (w529:string[])
            n307 = call-poly <vilib>:"NT Read Value.vi"("Default Value"=w529, "Name"="Legal_Actuator_Names") -> ("String Array"=w528:string[])  [unwired: 8 in, 1 out]
            n308 = call-poly <vilib>:"NT Write Value.vi"("String"=w527, "Name"="Test_Actuator_Name") -> ()  [unwired: 9 in, 1 out]
            n309 = call-poly <vilib>:"NT Write Value.vi"("Numeric"="Test_Actuator_Value", "Name"="Test_Actuator_Value") -> ()  [unwired: 9 in, 1 out]
            n310 = call-poly <vilib>:"NT Write Value.vi"("Numeric"="Test_Actuator_Period", "Name"="Test_Actuator_Period") -> ()  [unwired: 9 in, 1 out]
            n311 = property on="Actuator Testing" class="Ring (strict)"("Strings []"=w528) -> ()  [unwired: 2 in, 2 out]
          }
          frame #6 {
            w600 = "H" ("x")
            # "drivebase subsytem"
            n312 = call-poly <vilib>:"NT Read Value.vi"("Name"="Field_Oriented") -> ("Boolean"=→"Field_Oriented":bool)  [unwired: 9 in, 1 out]
            n313 = call-poly <vilib>:"NT Read Value.vi"("Name"="IMU_Failure") -> ("Boolean"=→"IMU_Failure":bool)  [unwired: 9 in, 1 out]
            n314 = call-poly <vilib>:"NT Read Value.vi"("Name"="Wheel_0S_Temp") -> ("Numeric"=→"Wheel_0S_Temp":dbl)  [unwired: 9 in, 1 out]
            n315 = call-poly <vilib>:"NT Read Value.vi"("Name"="Wheel_0_Azimuth") -> ("Numeric"=→"Wheel_0_Azimuth":dbl)  [unwired: 9 in, 1 out]
            n316 = call-poly <vilib>:"NT Read Value.vi"("Name"="Wheel_0S_Velocity") -> ("Numeric"=→"Wheel_0S_Velocity":dbl)  [unwired: 9 in, 1 out]
            n317 = call-poly <vilib>:"NT Read Value.vi"("Name"="Wheel_1S_Temp") -> ("Numeric"=→"Wheel_1S_Temp":dbl)  [unwired: 9 in, 1 out]
            n318 = call-poly <vilib>:"NT Read Value.vi"("Name"="Wheel_1_Azimuth") -> ("Numeric"=→"Wheel_1_Azimuth":dbl)  [unwired: 9 in, 1 out]
            n319 = call-poly <vilib>:"NT Read Value.vi"("Name"="Wheel_1S_Velocity") -> ("Numeric"=→"Wheel_1S_Velocity":dbl)  [unwired: 9 in, 1 out]
            n320 = call-poly <vilib>:"NT Read Value.vi"("Name"="Wheel_2S_Temp") -> ("Numeric"=→"Wheel_2S_Temp":dbl)  [unwired: 9 in, 1 out]
            n321 = call-poly <vilib>:"NT Read Value.vi"("Name"="Wheel_2_Azimuth") -> ("Numeric"=→"Wheel_2_Azimuth":dbl)  [unwired: 9 in, 1 out]
            n322 = call-poly <vilib>:"NT Read Value.vi"("Name"="Wheel_2S_Velocity") -> ("Numeric"=→"Wheel_2S_Velocity":dbl)  [unwired: 9 in, 1 out]
            n323 = call-poly <vilib>:"NT Read Value.vi"("Name"="Wheel_3S_Temp") -> ("Numeric"=→"Wheel_3S_Temp":dbl)  [unwired: 9 in, 1 out]
            n324 = call-poly <vilib>:"NT Read Value.vi"("Name"="Wheel_3_Azimuth") -> ("Numeric"=→"Wheel_3_Azimuth":dbl)  [unwired: 9 in, 1 out]
            n325 = call-poly <vilib>:"NT Read Value.vi"("Name"="Wheel_3S_Velocity") -> ("Numeric"=→"Wheel_3S_Velocity":dbl)  [unwired: 9 in, 1 out]
            n326 = call-poly <vilib>:"NT Read Value.vi"("Default Value"=bool[] [FALSE, FALSE, FALSE, FALSE], "Name"="Shifter_Faults") -> ("Boolean Array"=w626:bool[])  [unwired: 8 in, 1 out]
            "Shifter_Faults_Array" <- w626
            n327 = call-poly <vilib>:"NT Read Value.vi"("Name"="Drive_Overheat") -> ("Boolean Array"=w601:bool[])  [unwired: 9 in, 1 out]
            "Drive_Overheat_Array" <- w601
            n328 = call-poly <vilib>:"NT Read Value.vi"("Default Value"=string[] ["U", "U", "U", "U"], "Name"="Shifter_States") -> ("String Array"=w615:string[])  [unwired: 8 in, 1 out]
            n329 = call-poly <vilib>:"NT Read Value.vi"("Default Value"=bool[] [FALSE, FALSE, FALSE, FALSE], "Name"="Module_Faults") -> ("Boolean Array"=w558:bool[])  [unwired: 8 in, 1 out]
            "Azimuth_Error_Array" <- w558
            n330 = Index Array(array=w615) -> (element #1=w631:string, element #2=w632:string, element #3=w633:string, element #4=w634:string)  [unwired: 4 in]
            "Wheel_0_Shifter_State" <- w631
            "Wheel_1_Shifter_State" <- w632
            "Wheel_2_Shifter_State" <- w633
            "Wheel_3_Shifter_State" <- w634
            n331 = Index Array(array=w626) -> (element #1=w623:bool, element #2=w622:bool, element #3=w621:bool, element #4=w620:bool)  [unwired: 4 in]
            n332 = Or Array Elements(Boolean array=w558) -> (logical OR=→"Drive_Train_Azimuth":bool)
            n333 = Index Array(array=w601) -> (element #1=w614:bool, element #2=w608:bool, element #3=w607:bool, element #4=w606:bool)  [unwired: 4 in]
            n334 = Index Array(array=w558) -> (element #1=w627:bool, element #2=w628:bool, element #3=w629:bool, element #4=w630:bool)  [unwired: 4 in]
            n335 = Compound Arithmetic op=OR(w623, w622, w621, w620) -> (→"Drive_Train_Shifter":bool)
            n336 = Compound Arithmetic op=OR(w614, w608, w607, w606) -> (→"Drive_Train_Overheat":bool)
            n337 = Select(t=u32 16711680 ("Numeric Text.Text Colors:Text Color"), s=w623, f=u32 4934475 ("Numeric Text.Text Colors:Text Color")) -> (s? t:f=w616:u32)
            n338 = Equal?(x=w600, y=w631) -> (x = y?=→"High_Gear_0":bool)
            n339 = Equal?(x=w600, y=w632) -> (x = y?=→"High_Gear_1":bool)
            n340 = Equal?(x=w600, y=w633) -> (x = y?=→"High_Gear_2":bool)
            n341 = Equal?(x=w600, y=w634) -> (x = y?=→"High_Gear_3":bool)
            n342 = Select(t=u32 16711680 ("Numeric Text.Text Colors:Text Color"), s=w622, f=u32 4934475 ("Numeric Text.Text Colors:Text Color")) -> (s? t:f=w617:u32)
            n343 = Select(t=u32 16711680 ("Numeric Text.Text Colors:Text Color"), s=w621, f=u32 4934475 ("Numeric Text.Text Colors:Text Color")) -> (s? t:f=w618:u32)
            n344 = Select(t=u32 16711680 ("Numeric Text.Text Colors:Text Color"), s=w620, f=u32 4934475 ("Numeric Text.Text Colors:Text Color")) -> (s? t:f=w619:u32)
            n345 = Select(t=u32 16711680 ("Numeric Text.Text Colors:Text Color"), s=w627, f=u32 4934475 ("Numeric Text.Text Colors:Text Color")) -> (s? t:f=w610:u32)
            n346 = Select(t=u32 16711680 ("Numeric Text.Text Colors:Text Color"), s=w628, f=u32 4934475 ("Numeric Text.Text Colors:Text Color")) -> (s? t:f=w611:u32)
            n347 = Select(t=u32 16711680 ("Numeric Text.Text Colors:Text Color"), s=w614, f=u32 4934475 ("Numeric Text.Text Colors:Text Color")) -> (s? t:f=w602:u32)
            n348 = Select(t=u32 16711680 ("Numeric Text.Text Colors:Text Color"), s=w629, f=u32 4934475 ("Numeric Text.Text Colors:Text Color")) -> (s? t:f=w612:u32)
            n349 = Select(t=u32 16711680 ("Numeric Text.Text Colors:Text Color"), s=w630, f=u32 4934475 ("Numeric Text.Text Colors:Text Color")) -> (s? t:f=w613:u32)
            n350 = Select(t=u32 16711680 ("Numeric Text.Text Colors:Text Color"), s=w608, f=u32 4934475 ("Numeric Text.Text Colors:Text Color")) -> (s? t:f=w603:u32)
            n351 = Select(t=u32 16711680 ("Numeric Text.Text Colors:Text Color"), s=w607, f=u32 4934475 ("Numeric Text.Text Colors:Text Color")) -> (s? t:f=w604:u32)
            n352 = Select(t=u32 16711680 ("Numeric Text.Text Colors:Text Color"), s=w606, f=u32 4934475 ("Numeric Text.Text Colors:Text Color")) -> (s? t:f=w605:u32)
            n353 = property on="Wheel_0_Shifter_State" class="Str"("Text.BG Color"=w616) -> ()  [unwired: 2 in, 2 out]
            n354 = property on="Wheel_1_Shifter_State" class="Str"("Text.BG Color"=w617) -> ()  [unwired: 2 in, 2 out]
            n355 = property on="Wheel_2_Shifter_State" class="Str"("Text.BG Color"=w618) -> ()  [unwired: 2 in, 2 out]
            n356 = property on="Wheel_3_Shifter_State" class="Str"("Text.BG Color"=w619) -> ()  [unwired: 2 in, 2 out]
            n357 = property on="Wheel_0S_Temp" class="DigNum (strict)"("NumText.BG Color"=w602) -> ()  [unwired: 2 in, 2 out]
            n358 = property on="Wheel_1S_Temp" class="DigNum (strict)"("NumText.BG Color"=w603) -> ()  [unwired: 2 in, 2 out]
            n359 = property on="Wheel_2S_Temp" class="DigNum (strict)"("NumText.BG Color"=w604) -> ()  [unwired: 2 in, 2 out]
            n360 = property on="Wheel_3S_Temp" class="DigNum (strict)"("NumText.BG Color"=w605) -> ()  [unwired: 2 in, 2 out]
            n361 = property on="Wheel_0_Azimuth" class="DigNum (strict)"("NumText.BG Color"=w610) -> ()  [unwired: 2 in, 2 out]
            n362 = property on="Wheel_1_Azimuth" class="DigNum (strict)"("NumText.BG Color"=w611) -> ()  [unwired: 2 in, 2 out]
            n363 = property on="Wheel_2_Azimuth" class="DigNum (strict)"("NumText.BG Color"=w612) -> ()  [unwired: 2 in, 2 out]
            n364 = property on="Wheel_3_Azimuth" class="DigNum (strict)"("NumText.BG Color"=w613) -> ()  [unwired: 2 in, 2 out]
            n365 = local read "Legal_Drivers"() -> (w544:string[])
            n366 = local read "Driver Profile"() -> (w543:u16)
            n367 = And(x="Calibrate_Wheels", y="Arm_Calibrate") -> (x .and. y?=w565:bool)
            n368 = Not(x="Arm_Calibrate") -> (.not. x?=w568:bool)
            n369 = call-poly <vilib>:"NT Write Value.vi"("Boolean"="Zero_Wheels", "Name"="Zero_Wheels") -> ()  [unwired: 9 in, 1 out]
            n370 = call-poly <vilib>:"NT Write Value.vi"("Boolean"=w565, "Name"="Calibrate_Wheels") -> ()  [unwired: 9 in, 1 out]
            n371 = To Long Integer(number=w543) -> (32bit integer=w541:i32)
            n372 = Select(t=cluster{u32, u32}[] [{11776947, 16448250}, {16448250, 16448250}] ("Colors [4]"), s=w568, f=cluster{u32, u32}[] [{6618880, 16448250}, {16448250, 16448250}] ("Colors [4]")) -> (s? t:f=w567:cluster{u32, u32}[])
            n373 = Cluster To Array(cluster="New_Driver_Profile_Setpoints") -> (array=w551:dbl[])
            n374 = Index Array(array=w544, index=w541) -> (element=→"Current_Driver_Profile":string)
            n375 = call-poly <vilib>:"NT Read Value.vi"("Default Value"=dbl[] [0.0, 0.0, 0.0, 0.0, 0.0, 0.0], "Name"="Current_Driver_Profile_Setpoints") -> ("Numeric Array"=w549:dbl[])  [unwired: 8 in, 1 out]
            n376 = property on="Calibrate_Wheels" class="Bool"("Colors [4]"=w567) -> ()  [unwired: 2 in, 2 out]
            n377 = Array To Cluster(array=w549) -> (cluster=w545:T22)
            "Current_Driver_Profile_Setpoints" <- w545
            n378 = call-poly <vilib>:"NT Write Value.vi"("Numeric Array"=w551, "Name"="New_Driver_Profile_Setpoints") -> ()  [unwired: 9 in, 1 out]
            n379 = call-poly <vilib>:"NT Write Value.vi"("Boolean"="Apply_Driver_Profile_Setpoints", "Name"="Apply_Driver_Profile_Setpoints") -> ()  [unwired: 9 in, 1 out]
            n380 = feedback-in #3(w549) -> ()
            n381 = feedback #3(dbl[] [0.0, 0.0, 0.0, 0.0, 0.0, 0.0] ("Default Value")) -> (w548:dbl[])
            n382 = Not Equal?(x=w549, y=w548) -> (x != y?=w547:bool[])
            n383 = Or Array Elements(Boolean array=w547) -> (logical OR=w546:bool)
            n384 = case shown="False" w546 {
              tunnel: w545 -> [_ w667]
              frame False {
              }
              frame True {
                n385 = property on="New_Driver_Profile_Setpoints" class="Clust (strict)"("Value"=w667) -> ()  [unwired: 2 in, 2 out]
              }
            }
          }
          frame #7 {
            # "climber subsystem"
            # "ball handling subsystems"
            # "ball handling and climber subsystems"
            n386 = call-poly <vilib>:"NT Read Value.vi"("Name"="Intake_On") -> ("Boolean"=→"Intake_On":bool)  [unwired: 9 in, 1 out]
            n387 = call-poly <vilib>:"NT Read Value.vi"("Name"="Intake_Overheat") -> ("Boolean"=w678:bool)  [unwired: 9 in, 1 out]
            "Intake_Overheat" <- w678
            n388 = call-poly <vilib>:"NT Read Value.vi"("Name"="Intake_Temp") -> ("Numeric"=→"Intake_Temp":dbl)  [unwired: 9 in, 1 out]
            n389 = Select(t=u32 16711680 ("Numeric Text.Text Colors:Text Color"), s=w678, f=u32 4934475 ("Numeric Text.Text Colors:Text Color")) -> (s? t:f=w677:u32)
            n390 = property on="Intake_Temp" class="DigNum (strict)"("NumText.BG Color"=w677) -> ()  [unwired: 2 in, 2 out]
            n391 = call-poly <vilib>:"NT Read Value.vi"("Name"="Climber_Climbing") -> ("Boolean"=→"Climber_Climbing":bool)  [unwired: 9 in, 1 out]
          }
          frame #8 {
            # "shooter subsystem"
            n392 = call-poly <vilib>:"NT Read Value.vi"("Name"="Shooter_Spinning") -> ("Boolean"=→"Shooter_Spinning":bool)  [unwired: 9 in, 1 out]
            n393 = call-poly <vilib>:"NT Read Value.vi"("Name"="Out_Of_Range") -> ("Boolean"=→"Out_Of_Range":bool)  [unwired: 9 in, 1 out]
            n394 = call-poly <vilib>:"NT Read Value.vi"("Name"="Shooter_Firing") -> ("Boolean"=→"Shooter_Firing":bool)  [unwired: 9 in, 1 out]
            n395 = call-poly <vilib>:"NT Read Value.vi"("Name"="Pointed_At_Target") -> ("Boolean"=→"Pointed_At_Target":bool)  [unwired: 9 in, 1 out]
            n396 = call-poly <vilib>:"NT Read Value.vi"("Name"="Shooter_Ready") -> ("Boolean"=→"Shooter_Ready":bool)  [unwired: 9 in, 1 out]
            n397 = call-poly <vilib>:"NT Read Value.vi"("Default Value"=0.0, "Name"="Balls_Shot_Total") -> ("Numeric"=w763:dbl)  [unwired: 8 in, 1 out]
            n398 = call-poly <vilib>:"NT Read Value.vi"("Name"="Retrieved_Shooter_Power") -> ("Numeric"=→"Shooter_Power":dbl)  [unwired: 9 in, 1 out]
            n399 = call-poly <vilib>:"NT Read Value.vi"("Name"="Retrieved_Kicker_Power") -> ("Numeric"=→"Kicker_Power":dbl)  [unwired: 9 in, 1 out]
            n400 = call-poly <vilib>:"NT Read Value.vi"("Name"="Shooter_0_Speed (rpm)") -> ("Numeric"=w754:dbl)  [unwired: 9 in, 1 out]
            "Shooter_0_RPM_Actual_Detail" <- w754
            n401 = call-poly <vilib>:"NT Read Value.vi"("Name"="Shooter_1_Speed (rpm)") -> ("Numeric"=w755:dbl)  [unwired: 9 in, 1 out]
            "Shooter_1_RPM_Actual_Detail" <- w755
            n402 = call-poly <vilib>:"NT Read Value.vi"("Name"="Kicker_Speed (rpm)") -> ("Numeric"=→"Kicker_RPM_Actual_Detail":dbl)  [unwired: 9 in, 1 out]
            n403 = call-poly <vilib>:"NT Read Value.vi"("Name"="Shooter_Goal_Speed (rpm)") -> ("Numeric"=→"Shooter_RPM_Goal" →"Shooter_RPM_Goal_Detail":dbl)  [unwired: 9 in, 1 out]
            n404 = call-poly <vilib>:"NT Read Value.vi"("Name"="Kicker_Goal_Speed (rpm)") -> ("Numeric"=→"Kicker_RPM_Goal_Detail":dbl)  [unwired: 9 in, 1 out]
            n405 = call-poly <vilib>:"NT Read Value.vi"("Name"="Shooter_0_Temp (C)") -> ("Numeric"=→"Shooter_0_Temp":dbl)  [unwired: 9 in, 1 out]
            n406 = call-poly <vilib>:"NT Read Value.vi"("Name"="Shooter_1_Temp (C)") -> ("Numeric"=→"Shooter_1_Temp":dbl)  [unwired: 9 in, 1 out]
            n407 = call-poly <vilib>:"NT Read Value.vi"("Name"="Kicker_Temp (C)") -> ("Numeric"=→"Kicker_Temp":dbl)  [unwired: 9 in, 1 out]
            n408 = To Long Integer(number=w763) -> (32bit integer=→"Balls_Shot":i32)
            n409 = Compound Arithmetic op=ADD(w754, w755) -> (w756:dbl)
            n410 = Divide(x=w756, y=2.0) -> (x/y=→"Shooter_RPM_Actual":dbl)
            n411 = call-poly <vilib>:"NT Read Value.vi"("Name"="Beam_Break_Raw") -> ("Numeric"=w730:dbl)  [unwired: 9 in, 1 out]
            n412 = call-poly <vilib>:"NT Read Value.vi"("Name"="Cowl_State") -> ("String"=w733:string)  [unwired: 9 in, 1 out]
            n413 = call-poly <vilib>:"NT Read Value.vi"("Name"="LIDAR_Fault") -> ("Boolean"=→"LIDAR_Fault":bool)  [unwired: 9 in, 1 out]
            n414 = call-poly <vilib>:"NT Read Value.vi"("Name"="LIDAR_Distance_To_Target") -> ("Numeric"=→"LIDAR_Distance_To_Target":dbl)  [unwired: 9 in, 1 out]
            n415 = To Long Integer(number=w730) -> (32bit integer=→"Beam_Break_Raw":i32)
            n416 = case shown="\"A\", Default" w733 {
              tunnel: [0.0 1.0] -> w732
              frame "A", Default {
              }
              frame "B" {
              }
            }
            "Cowl_Position" <- w732
            n417 = call-poly <vilib>:"NT Read Value.vi"("Name"="Shoot_Overheat") -> ("Boolean Array"=w683:bool[])  [unwired: 9 in, 1 out]
            "Shooter_Overheat_Array" <- w683
            n418 = call-poly <vilib>:"NT Read Value.vi"("Name"="Shooter_Motor_Failure") -> ("Boolean Array"=w722:bool[])  [unwired: 9 in, 1 out]
            "Shooter_Motor_Failure_Array" <- w722
            n419 = Index Array(array=w683) -> (element #1=w720:bool, element #2=w719:bool, element #3=w729:bool)  [unwired: 3 in]
            n420 = Index Array(array=w722) -> (element #1=w726:bool, element #2=w725:bool)  [unwired: 2 in]
            n421 = Compound Arithmetic op=OR(w720, w719, w729) -> (→"Shooter_Overheat":bool)
            n422 = Select(t=u32 16711680 ("Numeric Text.Text Colors:Text Color"), s=w720, f=u32 4934475 ("Numeric Text.Text Colors:Text Color")) -> (s? t:f=w717:u32)
            n423 = Compound Arithmetic op=OR(w726, w725) -> (→"Shooter_Motor_Failure":bool)
            n424 = Select(t=u32 16711680 ("Numeric Text.Text Colors:Text Color"), s=w719, f=u32 4934475 ("Numeric Text.Text Colors:Text Color")) -> (s? t:f=w718:u32)
            n425 = Select(t=u32 16711680 ("Numeric Text.Text Colors:Text Color"), s=w729, f=u32 4934475 ("Numeric Text.Text Colors:Text Color")) -> (s? t:f=w728:u32)
            n426 = Select(t=u32 16711680 ("Numeric Text.Text Colors:Text Color"), s=w726, f=u32 4934475 ("Numeric Text.Text Colors:Text Color")) -> (s? t:f=w723:u32)
            n427 = Select(t=u32 16711680 ("Numeric Text.Text Colors:Text Color"), s=w725, f=u32 4934475 ("Numeric Text.Text Colors:Text Color")) -> (s? t:f=w724:u32)
            n428 = property on="Shooter_0_Temp" class="DigNum (strict)"("NumText.BG Color"=w717) -> ()  [unwired: 2 in, 2 out]
            n429 = property on="Shooter_1_Temp" class="DigNum (strict)"("NumText.BG Color"=w718) -> ()  [unwired: 2 in, 2 out]
            n430 = property on="Kicker_Temp" class="DigNum (strict)"("NumText.BG Color"=w728) -> ()  [unwired: 2 in, 2 out]
            n431 = property on="Shooter_0_RPM_Actual_Detail" class="DigNum (strict)"("NumText.BG Color"=w723) -> ()  [unwired: 2 in, 2 out]
            n432 = property on="Shooter_1_RPM_Actual_Detail" class="DigNum (strict)"("NumText.BG Color"=w724) -> ()  [unwired: 2 in, 2 out]
            n433 = Build Array("N/A") -> (w692:string[])
            n434 = call-poly <vilib>:"NT Read Value.vi"("Name"="Selected_Shooter_Setpoint_Value (rpm)") -> ("Numeric"=w680:dbl)  [unwired: 9 in, 1 out]
            "Selected_Shooter_Setpoint_Value (rpm)" <- w680
            n435 = To Double Precision Float(number="Selected_Shooter_Setpoint_Index") -> (double precision float=w689:dbl)
            n436 = call-poly <vilib>:"NT Read Value.vi"("Default Value"=w692, "Name"="Legal_Shooter_Setpoints") -> ("String Array"=w691:string[])  [unwired: 8 in, 1 out]
            n437 = call-poly <vilib>:"NT Write Value.vi"("Numeric"="New_Shooter_Setpoint (rpm)", "Name"="New_Shooter_Setpoint (rpm)") -> ()  [unwired: 9 in, 1 out]
            n438 = call-poly <vilib>:"NT Write Value.vi"("Boolean"="Apply_New_Shooter_Setpoint", "Name"="Apply_New_Shooter_Setpoint") -> ()  [unwired: 9 in, 1 out]
            n439 = call-poly <vilib>:"NT Write Value.vi"("Numeric"=w689, "Name"="Selected_Shooter_Setpoint_Index") -> ()  [unwired: 9 in, 1 out]
            n440 = property on="Selected_Shooter_Setpoint_Index" class="Ring (strict)"("Strings []"=w691) -> ()  [unwired: 2 in, 2 out]
            n441 = feedback-in #4(w680) -> ()
            n442 = feedback #4(0.0 ("Numeric")) -> (w681:dbl)
            n443 = Not Equal?(x=w681, y=w680) -> (x != y?=w679:bool)
            n444 = case shown="True" w679 {
              tunnel: w680 -> [_ w768]
              frame False {
              }
              frame True {
                n445 = property on="New_Shooter_Setpoint (rpm)" class="DigNum (strict)"("Value"=w768) -> ()  [unwired: 2 in, 2 out]
              }
            }
          }
          frame #9 {
            w776 = FALSE  # LIDAR
            w886 = FALSE  # Compressor
            w780 = FALSE
            w887 = FALSE  # LimeLight
            # "dynamic overlays"
            # "manage audible warnings"
            # "# of false elements"
            # "find # of trues"
            # "caution alarms"
            # "error management and driver assistance"
            n446 = local read "Shooter_Overheat_Array"() -> (w786:bool[])
            n447 = local read "Drive_Overheat_Array"() -> (w903:bool[])
            n448 = local read "Azimuth_Error_Array"() -> (w909:bool[])
            n449 = local read "Shooter_Motor_Failure_Array"() -> (w779:bool[])
            n450 = local read "Shifter_Faults_Array"() -> (w913:bool[])
            n451 = local read "Intake_Overheat"() -> (w902:bool)
            n452 = local read "CAN_Bus_Fault"() -> (w900:bool)
            n453 = local read "Battery_Critical"() -> (w895:bool)
            n454 = local read "Electrical_Fault"() -> (w896:bool)
            n455 = local read "Pressure_Vent"() -> (w899:bool)
            n456 = local read "IMU_Failure"() -> (w901:bool)
            n457 = local read "Slow_Loop"() -> (w897:bool)
            n458 = Index Array(array=w903) -> (element #1=w904:bool, element #2=w905:bool, element #3=w906:bool, element #4=w907:bool)  [unwired: 4 in]
            n459 = Index Array(array=w909) -> (element #1=w908:bool, element #2=w910:bool, element #3=w911:bool, element #4=w912:bool)  [unwired: 4 in]
            n460 = Index Array(array=w913) -> (element #1=w914:bool, element #2=w915:bool, element #3=w916:bool, element #4=w917:bool)  [unwired: 4 in]
            n461 = local read "Camera_1_Fault"() -> (w772:bool)
            n462 = local read "Camera_2_Fault"() -> (w773:bool)
            n463 = local read "Compressor_On"() -> (w898:bool)
            n464 = local read "Pressure_Leak"() -> (w774:bool)
            n465 = Index Array(array=w779) -> (element #1=w778:bool, element #2=w777:bool)  [unwired: 2 in]
            n466 = Index Array(array=w786) -> (element #1=w784:bool, element #2=w783:bool, element #3=w785:bool)  [unwired: 3 in]
            n467 = local read "LIDAR_Fault"() -> (w775:bool)
            n468 = Or(x=w772, y=w773) -> (x .or. y?=w771:bool)
            n469 = Or(x=w784, y=w778) -> (x .or. y?=w782:bool)
            n470 = Or(x=w783, y=w777) -> (x .or. y?=w781:bool)
            n471 = Build Array(w895, w896, w897, w887, w886, w899, w900, w901, w904, w905, w906, w907, w908, w910, w911, w912, w914, w915, w916, w917, w902, FALSE ("element"), w785, w782, w781, w776) -> (w802:bool[])
            n472 = Initialize Array(FALSE, 25 ("dimension size")) -> (w804:bool[])
            n473 = Build Array(w780, w780, w780, w771, w898, w774, w780, w780, w780, w780, w780, w780, w780, w780, w780, w780, w780, w780, w780, w780, w780, w780, w780, w780, w780, w775) -> (w803:bool[])
            n474 = local read "Hide_Popups"() -> (w894:bool)
            n475 = Build Array("Error_Help", "Driver_Help", "Manipulator_Help") -> (w789:bool[])
            n476 = Not(x=w894) -> (.not. x?=w799:bool)
            n477 = Or Array Elements(Boolean array=w789) -> (logical OR=w800:bool)
            n478 = And(x=w800, y=w799) -> (x .and. y?=w801:bool)
            n479 = Not(x=w800) -> (.not. x?=w808:bool)
            n480 = Build Array (concatenate)(w808, w789) -> (w807:bool[])
            n481 = property on="Help Graphic" class="ImageControl"("Visible"=w801) -> ()  [unwired: 2 in, 2 out]
            n482 = call "StateSelection.vi"("Disallowed States"=bool[] [FALSE, FALSE, FALSE, FALSE], "State Triggers"=w807, "State Names"=string[] ["No Help", "Error Help", "Driver Help", "Manipulator Help"]) -> ("Selected State"=w813:string)
            n483 = case shown="\"Error Help\"" w813 {
              tunnel: [_ w924 w925 w927] -> w805
              tunnel: w804 -> [_ w922 _ _]
              tunnel: w803 -> [_ w921 _ _]
              tunnel: w802 -> [_ w923 _ _]
              tunnel: w801 -> [_ w920 _ _]
              frame "No Help", Default {
              }
              frame "Error Help" {
                n484 = call "RenderRobotSystemsDiagram.vi"("Enable"=w920, "Cautions"=w921, "Nominals"=w922, "Alarms"=w923) -> ("Robot Systems Diagram"=w924:T3)  [unwired: 1 in]
              }
              frame "Driver Help" {
                n485 = call "RenderJoystickDiagram.vi"("Joystick Graphic Filename"="driver joystick diagram.png") -> ("Image Out"=w925:T3)  [unwired: 10 in]
              }
              frame "Manipulator Help" {
                n486 = call "RenderJoystickDiagram.vi"("Joystick Graphic Filename"="manipulator joystick diagram.png") -> ("Image Out"=w927:T3)  [unwired: 10 in]
              }
            }
            "Help Graphic" <- w805
            n487 = Or Array Elements(Boolean array=w789) -> (logical OR=w791:bool)
            n488 = Not(x=w791) -> (.not. x?=w790:bool)
            n489 = Or(x=w790, y=w789) -> (x .or. y?=w788:bool[])
            n490 = Index Array(array=w788, index #1=0 ("index")) -> (element #1=w794:bool, element #2=w793:bool, element #3=w792:bool)  [unwired: 2 in]
            n491 = Select(t=T16."Enabled" ("Disabled"), s=w792, f=T16."Disabled and Grayed Out" ("Disabled")) -> (s? t:f=w796:T16)
            n492 = Select(t=T16."Enabled" ("Disabled"), s=w794, f=T16."Disabled and Grayed Out" ("Disabled")) -> (s? t:f=w918:T16)
            n493 = Select(t=T16."Enabled" ("Disabled"), s=w793, f=T16."Disabled and Grayed Out" ("Disabled")) -> (s? t:f=w919:T16)
            n494 = property on="Error_Help" class="Bool (strict)"("DisabledEnum"=w918) -> ()  [unwired: 2 in, 2 out]
            n495 = property on="Driver_Help" class="Bool (strict)"("DisabledEnum"=w919) -> ()  [unwired: 2 in, 2 out]
            n496 = property on="Manipulator_Help" class="Bool (strict)"("DisabledEnum"=w796) -> ()  [unwired: 2 in, 2 out]
            n497 = local read "Master_Safety_Override_1"() -> (w851:bool)
            n498 = local read "Master_Safety_Override_2"() -> (w852:bool)
            n499 = local read "Arm_Calibrate_Joysticks"() -> (w869:bool)
            n500 = local read "Shooter_Motor_Failure"() -> (w864:bool)
            n501 = property on="Actuator Testing" class="Ring (strict)"() -> ("RingText.Text"=w853:string)  [unwired: 2 in, 2 out]
            n502 = local read "Drive_Train_Overheat"() -> (w857:bool)
            n503 = local read "Drive_Train_Azimuth"() -> (w859:bool)
            n504 = local read "Drive_Train_Shifter"() -> (w884:bool)
            n505 = local read "Shooter_Overheat"() -> (w863:bool)
            n506 = local read "Super_Test_Mode"() -> (w855:bool)
            n507 = local read "Auto_Test_Mode"() -> (w862:bool)
            n508 = local read "Intake_Overheat"() -> (w865:bool)
            n509 = local read "CAN_Bus_Fault"() -> (w870:bool)
            n510 = local read "Battery_Critical"() -> (w885:bool)
            n511 = local read "Electrical_Fault"() -> (w868:bool)
            n512 = local read "Arm_Calibrate"() -> (w860:bool)
            n513 = local read "Pressure_Vent"() -> (w858:bool)
            n514 = local read "IMU_Failure"() -> (w867:bool)
            n515 = local read "Slow_Loop"() -> (w856:bool)
            n516 = local read "Auto_Error"() -> (w861:bool)
            n517 = Not Equal?(x=w853, y="No_Test") -> (x != y?=w866:bool)
            n518 = And(x=w851, y=w852) -> (x .and. y?=w854:bool)
            n519 = Bundle(w854, "Super_Test_Mode"=w855, "Slow_Loop"=w856, "Drive_Train_Overheat"=w857, "Pressure_Vent"=w858, "Drive_Train_Azimuth"=w859, "Arm_Calibrate"=w860, "Auto_Error"=w861, "Auto_Test_Mode"=w862, "Shooter_Overheat"=w863, "Shooter_Motor_Failure"=w864, "Intake_Overheat"=w865, w866, "IMU_Failure"=w867, "Electrical_Fault"=w868, "Arm_Calibrate_Joysticks"=w869, "CAN_Bus_Fault"=w870, "Drive_Train_Shifter"=w884, "Battery_Critical"=w885) -> (w871:T23)  [unwired: 1 in]
            n520 = Cluster To Array(cluster=w871) -> (array=w876:bool[])
            n521 = call "BlinkLight.vi"() -> ("Blinked"=w850:bool)  [unwired: 1 in]
            n522 = Or Array Elements(Boolean array=w876) -> (logical OR=w882:bool)
            n523 = Select(t=w850, s=w882, f=FALSE) -> (s? t:f=w883:bool)
            "Master_Caution_1" <- w883
            "Master_Caution_0" <- w883
            "Master_Caution_2" <- w883
            n524 = Sort 1D Array(array=w876) -> (sorted array=w873:bool[])
            n525 = call-poly <vilib>:"NT Read Value.vi"("Name"="Robot_Mode") -> ("String"=w833:string)  [unwired: 9 in, 1 out]
            n526 = Search 1D Array(1D array=w873, element=TRUE, start index (0)=0) -> (index of element=w879:i32)
            n527 = call "EdgeTrigger.vi"("Input Signal"="Mute_Audible_Warnings") -> ("Rising Edge Trigger"=w840:bool)  [unwired: 2 out]
            n528 = Equal?(x=w833, y="Teleop Enabled") -> (x = y?=w834:bool)
            n529 = Array Size(array=w873) -> (size(s)=w875:i32)
            n530 = local read "Out_Of_Range"() -> (w821:bool)
            n531 = Equal?(x=w879, y=-1) -> (x = y?=w872:bool)
            n532 = call-poly <vilib>:"NT Write Value.vi"("Boolean"=w882, "Name"="Master_Caution") -> ()  [unwired: 9 in, 1 out]
            n533 = call-poly <vilib>:"NT Read Value.vi"("Name"="Power_Port_Target") -> ("Boolean"=w824:bool)  [unwired: 9 in, 1 out]
            n534 = call "EdgeTrigger.vi"("Input Signal"=w834) -> ("Rising Edge Trigger"=w835:bool)  [unwired: 2 out]
            n535 = Select(t=w875, s=w872, f=w879) -> (s? t:f=w874:i32)
            n536 = Subtract(x=w875, y=w874) -> (x-y=w878:i32)
            n537 = local read "Intake_On"() -> (→"Ret_Ball_Left" →"Ret_Ball_Right":bool)
            n538 = feedback #5(TRUE ("t")) -> (w838:bool)
            n539 = Not(x=w838) -> (.not. x?=w837:bool)
            n540 = Select(t=w837, s=w840, f=w838) -> (s? t:f=w832:bool)
            n541 = call-poly <vilib>:"NT Read Value.vi"("Name"="Feeder_Auto_Target") -> ("Boolean"=→"Ret_Feeder_Right" →"Ret_Feeder_Left":bool)  [unwired: 9 in, 1 out]
            n542 = call "BlinkLight.vi"() -> ("Blinked"=w818:bool)  [unwired: 1 in]
            n543 = Select(t=TRUE, s=w835, f=w832) -> (s? t:f=w836:bool)
            "Audible_Warnings_Enabled" <- w836
            n544 = feedback-in #5(w836) -> ()
            n545 = Number To Decimal String(number=w878) -> (decimal integer string=w877:string)  [unwired: 1 in]
            n546 = Select(t=w818, s=w821, f=TRUE) -> (s? t:f=w822:bool)
            n547 = Concatenate Strings("MASTER ALARM (" ("string"), w877, ")" ("string")) -> (w880:string)
            n548 = Select(t=w822, s=w824, f=FALSE) -> (s? t:f=→"Ret_Power_Port_Left" →"Ret_Power_Port_Right":bool)
            n549 = Select(t=w880, s=w883, f="") -> (s? t:f=w881:string)
            n550 = Select(t=cluster{u32, u32}[] [{6618880, 16448250}, {16448250, 16448250}] ("Colors [4]"), s=w836, f=cluster{u32, u32}[] [{16755474, 16448250}, {16448250, 16448250}] ("Colors [4]")) -> (s? t:f=w831:cluster{u32, u32}[])
            n551 = property on="Mute_Audible_Warnings" class="Bool"("Colors [4]"=w831) -> ()  [unwired: 2 in, 2 out]
            n552 = property on="Master_Caution_0" class="Bool (strict)"("BoolText.Text"=w881) -> ()  [unwired: 2 in, 2 out]
            n553 = property on="Master_Caution_1" class="Bool (strict)"("BoolText.Text"=w881) -> ()  [unwired: 2 in, 2 out]
            n554 = property on="Master_Caution_2" class="Bool (strict)"("BoolText.Text"=w881) -> ()  [unwired: 2 in, 2 out]
          }
        }
      }
    }
  }
  n555 = control-ref of="Test Tree"() -> (w37:refnum<vi>)
  n556 = call "InitChecklistCustom.vi"("ListBox in"=w1) -> ()  [unwired: 1 in]
  n557 = vi-ref "Playback Controls.vi"() -> (w33:refnum<vi>)
  n558 = control-ref of="Command Params"() -> (w15:refnum<vi>)
  n559 = while {
    tunnel: [w938] -> _
    tunnel: w37 -> [w937]
    tunnel: w33 -> [w936]
    tunnel: w32 -> [w935]
    tunnel: w31 -> [_]
    tunnel: w27 -> [w934]
    tunnel: w16 -> [w933]
    tunnel: w15 -> [w932]
    shift-right: [w931] -> _
    shift-left: _ -> [w930]
    tunnel: w14 -> [w929]
    i -> [w938]
    stop <- FALSE stop-if-true
    n560 = event shown="[9] \"CheckList\": Double Click" {
      selector: w935 -> [_ _ _ _ _ _ _ _ _ _ _ _ _ _ _ _ _ _ _ _ _]
      dyn-events: [_ _ _ _ _ _ _ _ _ _ _ _ _ _ _ _ w1196 _ _ _ _] -> _
      timeout: u32 60 ("milliseconds to wait") -> [_ _ _ _ _ _ _ _ _ _ _ _ _ _ _ _ _ _ _ _ _]
      tunnel: w937 -> [w950 _ _ _ _ _ _ _ _ _ _ _ _ _ _ _ _ _ _ _ _]
      tunnel: "Test Tree" -> [_ _ _ _ _ _ _ _ _ _ _ w1165 w1173 w1175 w1179 w1187 _ _ _ _ _]
      tunnel: w936 -> [_ _ _ _ _ _ _ _ _ _ _ _ _ _ _ _ w1198 _ w1216 _ _]
      tunnel: w934 -> [_ _ _ _ _ _ _ _ _ _ _ _ _ _ _ _ w1194 _ _ _ _]
      tunnel: w933 -> [_ _ _ _ _ _ _ _ _ _ _ _ _ _ _ _ w1192 _ _ _ _]
      tunnel: w932 -> [w945 _ _ _ _ _ w1116 _ _ _ _ _ _ _ _ _ _ _ _ _ _]
      tunnel: [w944 w993 w1095 w1100 w1109 w1113 w1114 w1123 w1133 w1140 w1152 w1164 w1171 w1174 w1178 w1186 w1191 w1211 w1213 w1217 w1230] -> w931
      tunnel: w930 -> [w944 w993 w1095 w1100 w1109 w1113 w1114 _ _ w1140 w1152 w1164 w1171 w1174 w1178 w1186 w1191 w1211 w1213 w1217 w1230]
      tunnel: w929 -> [w942 _ _ _ _ _ _ _ _ _ _ _ _ _ _ _ _ _ _ _ _]
      event Timeout {
        n561 = event-data() -> ()  [unwired: 1 in, 1 out]
        n562 = local read "Mode"() -> (w947:T7)
        n563 = case shown="\"Commands\"" "Dashboard Tab" {
          tunnel: w950 -> [_ _ w966 _ _]
          tunnel: "TestMode/Automatic/" ("Name Pattern") -> [_ _ w965 _ _]
          tunnel: T24 [{"Operation"=enum."Clear", "Color Box"=14013909}, {"Operation"=enum."Clear", "Color Box"=14013909}, {"Operation"=enum."Clear", "Color Box"=14013909}, {"Operation"=enum."Clear", "Color Box"=14013909}, {"Operation"=enum."Update", "Color Box"=14013909}, {"Operation"=enum."Update", "Color Box"=16777215}, {"Operation"=enum."Clear", "Color Box"=14013909}, {"Operation"=enum."Clear", "Color Box"=14013909}, {"Operation"=enum."Clear", "Color Box"=14013909}] -> [_ _ w958 _ w986]
          tunnel: w947 -> [_ _ w957 _ w985]
          tunnel: u32[] [15790320, 15790320, 15790320, 15790320, 16777215, 16777215, 15790320, 15790320, 15790320] -> [_ _ _ _ w991]
          tunnel: w945 -> [_ _ _ _ w979]
          tunnel: w942 -> [_ w952 _ _ _]
          frame "TeleOp", Default {
          }
          frame "Tune" {
            n564 = call <vilib>:"WPI_DashboardUpdateNames.vi"("Controls on Tab"=w952) -> ()  [unwired: 11 in]
          }
          frame "Test" {
            w964 = -2 ("Active Item:Row Number")
            n565 = Index Array(array=w958, index=w957) -> (element=w959:T27)
            n566 = Unbundle(w959) -> ("Operation"=w960:enum16{"Update", "Clear"}, "Color Box"=w961:u32)
            n567 = call <vilib>:"NT Read String.vi"("Name"="TestMode/TestName") -> ("String"=w955:string)  [unwired: 9 in, 1 out]
            n568 = call <vilib>:"NT Read and Format Entries as Tree.vi"("Operation"=w960, "Name Pattern"=w965, "Tree Refnum"=w966) -> ()  [unwired: 7 in, 2 out]
            n569 = case shown="\"\"" w955 {
              tunnel: "TestMode/TestProgress" ("Name") -> [w968 _]
              tunnel: "TestMode/TestProgressText" ("Name") -> [w967 _]
              frame Default {
                n570 = call <vilib>:"NT Read Number.vi"("Name"=w968) -> ("Numeric"=w969:dbl)  [unwired: 9 in, 1 out]
                n571 = call <vilib>:"NT Read String.vi"("Name"=w967) -> ("String"=w970:string)  [unwired: 9 in, 1 out]
                n572 = Bundle("Numeric"=w969, "String"=w970) -> (→"Progress":cluster{"Numeric":dbl, "String":string})  [unwired: 1 in]
              }
              frame "" {
                n573 = property on="Progress" class="Clust (strict)"("Visible"=FALSE) -> ()  [unwired: 2 in, 2 out]
                n574 = local write "Test Name"(u16 0) -> ()
              }
            }
            n575 = property on="Test Tree" class="Tree (strict)"("Active Item Row Number"=w964, "ActiveColNum"=w964, "CellBG"=w961, "Active Item Row Number"=-1 ("Active Item:Row Number"), "CellBG"=u32 5789784 ("Color Box")) -> ()  [unwired: 2 in, 2 out]
          }
          frame "Variables" {
            w976 = string[] ["CameraPublisher", "Usage", "DB"]  # Items to initially close
            n576 = First Call?() -> (First Call?: T/F=w977:bool)
            n577 = control-ref of="Tree"() -> (w978:refnum<vi>)
            n578 = Select(t=w976, s=w977, f=string[] []) -> (s? t:f=w974:string[])
            n579 = call <vilib>:"NT Read and Format Entries as Tree.vi"("Tags to  Close"=w974, "Tree Refnum"=w978) -> ()  [unwired: 8 in, 2 out]
          }
          frame "Commands" {
            w987 = u32 5789784 ("Color Box")
            w988 = T28 {"Row"=-1, "Column"=-2} ("Active Cell:Active Cell")
            w990 = T28 {"Row"=-2, "Column"=-2} ("Active Cell:Active Cell")
            n580 = Index Array(array=w991, index=w985) -> (element=w989:u32)
            n581 = Index Array(array=w986, index=w985) -> (element=w984:T27)
            n582 = Unbundle(w984) -> ("Operation"=w983:enum16{"Update", "Clear"})  [unwired: 1 out]
            n583 = local read "Command Selection"() -> (w982:i32)
            n584 = property on="Command Selection" class="MCListbox (strict)"("ActiveCell"=w990, "CellBG"=w989, "ActiveCell"=w988, "CellBG"=w987) -> ()  [unwired: 2 in, 2 out]
            n585 = call <vilib>:"WPI_DashboardUpdate RPC Info.vi"("Operation"=w983) -> ("update"=w981:bool, "commands"=w980:string[][])  [unwired: 9 in]
            n586 = property on="Command Selection" class="MCListbox (strict)"("ItemNames"=w980) -> ()  [unwired: 2 in, 2 out]
            n587 = property on="Command Params" class="Tbl (strict)"("Active Cell"=w990, "Cell BG Color"=w989, "Active Cell"=w988, "Cell BG Color"=w987) -> ()  [unwired: 2 in, 2 out]
            n588 = call <vilib>:"WPI_DashboardUpdate Command Params.vi"("Update"=w981, "NewVal"=w982, "Commands"=w980, "Param Tbl"=w979) -> ()  [unwired: 7 in, 1 out]
          }
        }
        n589 = call <vilib>:"Connextion Info.vi"() -> ("Connected"=→"NT Connection":bool)  [unwired: 10 in, 1 out]
      }
      event "Test Tree": Value Change {
        # "Show appropriate\ncontrols"
        n590 = event-data() -> ("CtlRef"=w996:refnum<vi>, "NewVal"=w994:string)  [unwired: 1 in]
        n591 = call <vilib>:"WPI_UtilitiesGetTreeIOName.vi"("NewVal"=w994, "TreeControl in"=w996) -> ("I/O Name"=w997:string)  [unwired: 9 in]
        n592 = case shown="\"Analog Out\", \"Motor\", \"PWM\"" w997 {
          selector: w997 -> [_ w1004 _ w1026 w1035 _]
          tunnel: w994 -> [_ _ w1023 w1025 _ w1042]
          tunnel: cluster{string[]}[] [{["640x480", "320x240", "160x120"]}, {["Auto", "Fixed indoor", "Fixed outdoor 1", "Fixed outdoor 2", "Fixed fluorescent 1", "Fixed fluorescent 2", "Hold current"]}, {["Auto", "Flicker-free 50 Hz", "Flicker-free 60 Hz", "Hold current"]}, {["None", "Prioritize frame rate", "Prioritize image quality"]}, {["Monochrome", "Color"]}] -> [_ _ _ _ _ w1041]
          frame Default {
            w999 = FALSE ("Visible")
            w998 = FALSE ("Visible")
            n593 = property on="Motor" class="Clust (strict)"("Visible"=w998) -> ()  [unwired: 2 in, 2 out]
            n594 = property on="Test Ring" class="Ring (strict)"("Visible"=w998) -> ()  [unwired: 2 in, 2 out]
            n595 = property on="Rev/Fwd" class="Clust (strict)"("Visible"=w999) -> ()  [unwired: 2 in, 2 out]
            n596 = property on="On/Off" class="Bool (strict)"("Visible"=w999) -> ()  [unwired: 2 in, 2 out]
            n597 = property on="Test Slider" class="Slide (strict)"("Visible"=w999) -> ()  [unwired: 2 in, 2 out]
          }
          frame "Analog Out", "Motor", "PWM" {
            w1005 = FALSE ("Visible")
            n598 = case shown="\"Analog Out\"" w1004 {
              tunnel: [1.0 ("Value") -1.0 ("Value") 0.0 ("Value")] -> w1003
              tunnel: [255.0 ("Value") 1.0 ("Value") 5.0 ("Value")] -> w1002
              tunnel: [128.0 ("Value") 0.0 ("Value") 0.0 ("Value")] -> w1001
              tunnel: [64.0 ("Value") 0.5 ("Value") 1.0 ("Value")] -> w1000
              frame "PWM" {
              }
              frame "Motor", Default {
              }
              frame "Analog Out" {
              }
            }
            n599 = property on="Motor" class="Clust (strict)"("Visible"=TRUE) -> ()  [unwired: 2 in, 2 out]
            n600 = property on="Value" class="Slide (strict)"("Value"=w1001, "Scale.Minimum"=w1003, "Scale.Maximum"=w1002, "Scale.Increment"=w1000) -> ()  [unwired: 2 in, 2 out]
            n601 = property on="On/Off" class="Bool (strict)"("Visible"=w1005) -> ()  [unwired: 2 in, 2 out]
            n602 = property on="Test Slider" class="Slide (strict)"("Visible"=w1005) -> ()  [unwired: 2 in, 2 out]
            n603 = property on="Test Ring" class="Ring (strict)"("Visible"=w1005) -> ()  [unwired: 2 in, 2 out]
            n604 = property on="Rev/Fwd" class="Clust (strict)"("Visible"=w1005) -> ()  [unwired: 2 in, 2 out]
          }
          frame "Servo" {
            w1021 = FALSE ("Visible")
            n605 = call <vilib>:"NT Read Number.vi"("Name"=w1023) -> ("Numeric"=w1022:dbl)  [unwired: 9 in, 1 out]
            n606 = property on="Test Slider" class="Slide (strict)"("Visible"=TRUE, "Scale.Maximum"=170.0 ("Scale.Range:Maximum")) -> ()  [unwired: 2 in, 2 out]
            n607 = local write "Test Slider"(w1022) -> ()
            n608 = property on="Motor" class="Clust (strict)"("Visible"=w1021) -> ()  [unwired: 2 in, 2 out]
            n609 = property on="Rev/Fwd" class="Clust (strict)"("Visible"=w1021) -> ()  [unwired: 2 in, 2 out]
            n610 = property on="On/Off" class="Bool (strict)"("Visible"=w1021) -> ()  [unwired: 2 in, 2 out]
            n611 = property on="Test Ring" class="Ring (strict)"("Visible"=w1021) -> ()  [unwired: 2 in, 2 out]
          }
          frame "Relay", "Solenoid" {
            w1024 = FALSE ("Visible")
            n612 = property on="Motor" class="Clust (strict)"("Visible"=w1024) -> ()  [unwired: 2 in, 2 out]
            n613 = property on="Test Slider" class="Slide (strict)"("Visible"=w1024) -> ()  [unwired: 2 in, 2 out]
            n614 = Search and Replace String(input string=w1025, search string="/Value  **", replace string="/Direction") -> (result string=w1031:string)  [unwired: 5 in, 3 out]
            n615 = property on="Test Ring" class="Ring (strict)"("Visible"=w1024) -> ()  [unwired: 2 in, 2 out]
            n616 = call <vilib>:"NT Read String.vi"("Name"=w1031) -> ("String"=w1029:string)  [unwired: 9 in, 1 out]
            n617 = Equal?(x="Both directions", y=w1029) -> (x = y?=w1027:bool)
            n618 = Not(x=w1027) -> (.not. x?=w1028:bool)
            n619 = property on="Rev/Fwd" class="Clust (strict)"("Visible"=w1027) -> ()  [unwired: 2 in, 2 out]
            n620 = property on="On/Off" class="Bool (strict)"("Visible"=w1028, "Caption.Text"=w1026) -> ()  [unwired: 2 in, 2 out]
          }
          frame "Compressor", "Digital Out" {
            w1034 = FALSE ("Visible")
            # "Get direction and finish"
            n621 = property on="Motor" class="Clust (strict)"("Visible"=w1034) -> ()  [unwired: 2 in, 2 out]
            n622 = property on="Test Slider" class="Slide (strict)"("Visible"=w1034) -> ()  [unwired: 2 in, 2 out]
            n623 = property on="Test Ring" class="Ring (strict)"("Visible"=w1034) -> ()  [unwired: 2 in, 2 out]
            n624 = property on="On/Off" class="Bool (strict)"("Visible"=TRUE, "Caption.Text"=w1035) -> ()  [unwired: 2 in, 2 out]
            n625 = property on="Rev/Fwd" class="Clust (strict)"("Visible"=FALSE) -> ()  [unwired: 2 in, 2 out]
          }
          frame "Camera" {
            n626 = call <vilib>:"Get Last Path Segment.vi"("String in"=w1042) -> ("String out"=w1043:string)  [unwired: 10 in]
            n627 = property on="On/Off" class="Bool (strict)"("Visible"=FALSE) -> ()  [unwired: 2 in, 2 out]
            n628 = property on="Motor" class="Clust (strict)"("Visible"=FALSE) -> ()  [unwired: 2 in, 2 out]
            n629 = property on="Rev/Fwd" class="Clust (strict)"("Visible"=FALSE) -> ()  [unwired: 2 in, 2 out]
            n630 = case shown="\"White Balance  **\"" w1043 {
              tunnel: w1042 -> [w1049 w1058 w1067 w1076 w1085 _ w1091]
              tunnel: w1041 -> [w1047 w1055 w1064 w1073 w1082 _ _]
              frame "Size  **" {
                n631 = Index Array(array=w1047) -> (element=w1046:cluster{string[]})  [unwired: 1 in]
                n632 = call <vilib>:"NT Read String.vi"("Name"=w1049) -> ("String"=w1048:string)  [unwired: 9 in, 1 out]
                n633 = Unbundle(w1046) -> (w1044:string[])
                n634 = Match First String(2:w1044, 3:w1048) -> (0:w1045:i32)  [unwired: 1 out]
                n635 = property on="Test Ring" class="Ring (strict)"("Value"=w1045, "Strings []"=w1044) -> ()  [unwired: 2 in, 2 out]
                n636 = property on="Test Ring" class="Ring (strict)"("Visible"=TRUE) -> ()  [unwired: 2 in, 2 out]
                n637 = property on="Test Slider" class="Slide (strict)"("Visible"=FALSE) -> ()  [unwired: 2 in, 2 out]
              }
              frame "White Balance  **" {
                n638 = Index Array(array=w1055, index=1) -> (element=w1056:cluster{string[]})
                n639 = call <vilib>:"NT Read String.vi"("Name"=w1058) -> ("String"=w1057:string)  [unwired: 9 in, 1 out]
                n640 = Unbundle(w1056) -> (w1053:string[])
                n641 = Match First String(2:w1053, 3:w1057) -> (0:w1052:i32)  [unwired: 1 out]
                n642 = property on="Test Ring" class="Ring (strict)"("Value"=w1052, "Strings []"=w1053) -> ()  [unwired: 2 in, 2 out]
                n643 = property on="Test Ring" class="Ring (strict)"("Visible"=TRUE) -> ()  [unwired: 2 in, 2 out]
                n644 = property on="Test Slider" class="Slide (strict)"("Visible"=FALSE) -> ()  [unwired: 2 in, 2 out]
              }
              frame "Exposure  **" {
                n645 = Index Array(array=w1064, index=2) -> (element=w1065:cluster{string[]})
                n646 = call <vilib>:"NT Read String.vi"("Name"=w1067) -> ("String"=w1066:string)  [unwired: 9 in, 1 out]
                n647 = Unbundle(w1065) -> (w1061:string[])
                n648 = Match First String(2:w1061, 3:w1066) -> (0:w1062:i32)  [unwired: 1 out]
                n649 = property on="Test Ring" class="Ring (strict)"("Value"=w1062, "Strings []"=w1061) -> ()  [unwired: 2 in, 2 out]
                n650 = property on="Test Ring" class="Ring (strict)"("Visible"=TRUE) -> ()  [unwired: 2 in, 2 out]
                n651 = property on="Test Slider" class="Slide (strict)"("Visible"=FALSE) -> ()  [unwired: 2 in, 2 out]
              }
              frame "Exposure Priority  **" {
                n652 = Index Array(array=w1073, index=3) -> (element=w1074:cluster{string[]})
                n653 = call <vilib>:"NT Read String.vi"("Name"=w1076) -> ("String"=w1075:string)  [unwired: 9 in, 1 out]
                n654 = Unbundle(w1074) -> (w1070:string[])
                n655 = Match First String(2:w1070, 3:w1075) -> (0:w1071:i32)  [unwired: 1 out]
                n656 = property on="Test Ring" class="Ring (strict)"("Value"=w1071, "Strings []"=w1070) -> ()  [unwired: 2 in, 2 out]
                n657 = property on="Test Ring" class="Ring (strict)"("Visible"=TRUE) -> ()  [unwired: 2 in, 2 out]
                n658 = property on="Test Slider" class="Slide (strict)"("Visible"=FALSE) -> ()  [unwired: 2 in, 2 out]
              }
              frame "Color Enable  **" {
                n659 = Index Array(array=w1082, index=4) -> (element=w1083:cluster{string[]})
                n660 = call <vilib>:"NT Read String.vi"("Name"=w1085) -> ("String"=w1084:string)  [unwired: 9 in, 1 out]
                n661 = Unbundle(w1083) -> (w1079:string[])
                n662 = Match First String(2:w1079, 3:w1084) -> (0:w1080:i32)  [unwired: 1 out]
                n663 = property on="Test Ring" class="Ring (strict)"("Value"=w1080, "Strings []"=w1079) -> ()  [unwired: 2 in, 2 out]
                n664 = property on="Test Ring" class="Ring (strict)"("Visible"=TRUE) -> ()  [unwired: 2 in, 2 out]
                n665 = property on="Test Slider" class="Slide (strict)"("Visible"=FALSE) -> ()  [unwired: 2 in, 2 out]
              }
              frame Default {
                n666 = property on="Test Ring" class="Ring (strict)"("Visible"=FALSE) -> ()  [unwired: 2 in, 2 out]
                n667 = property on="Test Slider" class="Slide (strict)"("Visible"=FALSE) -> ()  [unwired: 2 in, 2 out]
              }
              frame "Brightness  **", "Color Level  **", "Compression  **", "FPS  **", "Sharpness  **" {
                n668 = call <vilib>:"NT Read Number.vi"("Name"=w1091) -> ("Numeric"=w1090:dbl)  [unwired: 9 in, 1 out]
                n669 = local write "Test Slider"(w1090) -> ()
                n670 = property on="Test Slider" class="Slide (strict)"("Visible"=TRUE, "Scale.Maximum"=100.0 ("Scale.Range:Maximum")) -> ()  [unwired: 2 in, 2 out]
                n671 = property on="Test Ring" class="Ring (strict)"("Visible"=FALSE) -> ()  [unwired: 2 in, 2 out]
              }
            }
          }
        }
        n672 = property on="Progress" class="Clust (strict)"("Visible"=FALSE) -> ()  [unwired: 2 in, 2 out]
      }
      event "Test Name": Mouse Enter {
        # "Populate the ring with the list of tests"
        n673 = event-data() -> ()  [unwired: 1 in, 1 out]
        n674 = call <vilib>:"NT Read String Array.vi"("Name"="TestMode/TestList") -> ("String Array"=w1099:string[])  [unwired: 9 in, 1 out]
        n675 = Build Array (concatenate)("Select the test to run...", w1099) -> (w1098:string[])
        n676 = property on="Test Name" class="Ring (strict)"("Strings []"=w1098) -> ()  [unwired: 2 in, 2 out]
      }
      event "Test Name": Value Change {
        w1101 = FALSE ("Visible")
        # "Tell the robot the test name to run"
        n677 = event-data() -> ("NewVal"=w1105:u16)  [unwired: 1 in]
        n678 = property on="Test Name" class="Ring (strict)"() -> ("Strings []"=w1106:string[])  [unwired: 2 in, 2 out]
        n679 = local write "Progress"(T8 {"Test Progress"=0, "Test Progress Text"=""} ("Progress")) -> ()
        n680 = Index Array(array=w1106, index=w1105) -> (element=w1104:string)
        n681 = call <vilib>:"NT Write String.vi"("String"=w1104, "Name"="TestMode/TestName") -> ()  [unwired: 9 in, 1 out]
        n682 = property on="Progress" class="Clust (strict)"("Visible"=TRUE) -> ()  [unwired: 2 in, 2 out]
        n683 = property on="Motor" class="Clust (strict)"("Visible"=w1101) -> ()  [unwired: 2 in, 2 out]
        n684 = property on="Test Slider" class="Slide (strict)"("Visible"=w1101) -> ()  [unwired: 2 in, 2 out]
        n685 = property on="On/Off" class="Bool (strict)"("Visible"=w1101) -> ()  [unwired: 2 in, 2 out]
        n686 = property on="Rev/Fwd" class="Clust (strict)"("Visible"=w1101) -> ()  [unwired: 2 in, 2 out]
        n687 = property on="Test Ring" class="Ring (strict)"("Visible"=w1101) -> ()  [unwired: 2 in, 2 out]
      }
      event "Select Auto": Mouse Enter {
        # "Populate the combo box with the list of autonomous options"
        n688 = event-data() -> ()  [unwired: 1 in, 1 out]
        n689 = call <vilib>:"NT Read String Array.vi"("Name"="Auto List") -> ("String Array"=w1108:string[])  [unwired: 9 in, 1 out]
        n690 = property on="Select Auto" class="CmbBox"("Strings[]"=w1108) -> ()  [unwired: 2 in, 2 out]
      }
      event "Select Auto": Value Change {
        # "User modified the Auto Selection. Write to NT variable so robot knows."
        n691 = event-data() -> ("NewVal"=w1111:string)  [unwired: 1 in]
        n692 = call <vilib>:"NT Write String.vi"("String"=w1111, "Name"="Auto Selector") -> ()  [unwired: 9 in, 1 out]
      }
      event "Command Selection": Value Change {
        # "Get the params and show in table"
        n693 = event-data() -> ("NewVal"=w1117:i32)  [unwired: 1 in]
        n694 = property on="Command Selection" class="MCListbox (strict)"() -> ("ItemNames"=w1115:string[][])  [unwired: 2 in, 2 out]
        n695 = call <vilib>:"WPI_DashboardUpdate Command Params.vi"("NewVal"=w1117, "Commands"=w1115, "Param Tbl"=w1116) -> ()  [unwired: 8 in, 1 out]
      }
      event "Execute Command": Value Change {
        # "Started one, Unique ID holds\nresponse"
        n696 = event-data() -> ()  [unwired: 1 in, 1 out]
        n697 = property on="Command Selection" class="MCListbox (strict)"() -> ("ItemNames"=w1128:string[][])  [unwired: 2 in, 2 out]
        n698 = Index Array(array=w1128, index (row)="Command Selection", index (col)=0) -> (element=w1126:string)
        n699 = call <vilib>:"Invoke Commands.vi"("Command Params"="Command Params", "Function Name"=w1126) -> ("Params"=w1122:u8, "Started"=w1121:bool)  [unwired: 7 in, 1 out]
        n700 = Array Subset(array="Command Params", length (row)=w1122) -> (w1123:string[][])  [unwired: 3 in]
        n701 = Select(t="Executing" ("Cmd Status"), s=w1121, f="" ("Cmd Status")) -> (s? t:f=→"Cmd Status":string)
      }
      event "Command Selection": Double Click {
        n702 = event-data() -> ("Row"=w1136:i32)  [unwired: 1 in]
        n703 = property on="Command Selection" class="MCListbox (strict)"() -> ("ItemNames"=w1139:string[][])  [unwired: 2 in, 2 out]
        n704 = local read "Command Params"() -> (w1135:string[][])
        n705 = Index Array(array=w1139, index (row)=w1136, index (col)=0) -> (element=w1137:string)
        n706 = call <vilib>:"Invoke Commands.vi"("Command Params"=w1135, "Function Name"=w1137) -> ("Params"=w1134:u8, "Started"=w1129:bool)  [unwired: 7 in, 1 out]
        n707 = Array Subset(array=w1135, length (row)=w1134) -> (w1133:string[][])  [unwired: 3 in]
        n708 = Select(t="Executing" ("Cmd Status"), s=w1129, f="" ("Cmd Status")) -> (s? t:f=w1130:string)
        n709 = local write "Cmd Status"(w1130) -> ()
      }
      event "CheckList": Double Click {
        # "Shift clears all"
        # "Update symbols on the listbox"
        n710 = event-data() -> ("PlatMods.Shift"=w1141:bool, "Row"=w1143:i32)  [unwired: 1 in]
        n711 = case shown="True" w1141 {
          tunnel: w1143 -> [w1147 _]
          tunnel: 1 -> [w1146 _]
          frame False {
            n712 = property on="CheckList" class="LstBox (strict)"() -> ("Item Symbols"=w1145:i32[])  [unwired: 2 in, 2 out]
            n713 = Replace Array Subset(array=w1145, new element=w1146, index=w1147) -> (w1144:i32[])
            n714 = property on="CheckList" class="LstBox (strict)"("Item Symbols"=w1144) -> ()  [unwired: 2 in, 2 out]
          }
          frame True {
            w1148 = 0 ("Top Row")
            n715 = property on="CheckList" class="LstBox (strict)"() -> ("Number of Rows"=w1150:u32)  [unwired: 2 in, 2 out]
            n716 = Initialize Array(0, w1150) -> (w1149:i32[])
            n717 = property on="CheckList" class="LstBox (strict)"("Top Row"=w1148, "Value"=w1148, "Item Symbols"=w1149) -> ()  [unwired: 2 in, 2 out]
          }
        }
      }
      event "CheckList": Key Down {
        # "Update symbols on the listbox\nLeft and right keys check and uncheck"
        n718 = event-data() -> ("VKey"=w1154:T25)  [unwired: 1 in]
        n719 = case shown="\"Left\", \"Right\"" w1154 {
          selector: w1154 -> [w1159 _]
          tunnel: eventvkey."Left" ("VKey") -> [w1157 _]
          frame "Left", "Right" {
            n720 = Equal?(x=w1157, y=w1159) -> (x = y?=w1158:bool)
            n721 = Select(t=0, s=w1158, f=1) -> (s? t:f=w1160:i32)
            n722 = property on="CheckList" class="LstBox (strict)"() -> ("Item Symbols"=w1163:i32[])  [unwired: 2 in, 2 out]
            n723 = Replace Array Subset(array=w1163, new element=w1160, index="CheckList") -> (w1162:i32[])
            n724 = property on="CheckList" class="LstBox (strict)"("Item Symbols"=w1162) -> ()  [unwired: 2 in, 2 out]
          }
          frame Default {
          }
        }
      }
      event "Motor.Enable": Value Change {
        # "When the test mode otor enable helper is set, update that\ntree row item's value"
        n725 = event-data() -> ("NewVal"=w1169:bool)  [unwired: 1 in]
        n726 = Unbundle("Motor") -> ("Value"=w1168:dbl)  [unwired: 1 out]
        n727 = Select(t=w1168, s=w1169, f=0.0) -> (s? t:f=w1166:dbl)
        n728 = call <vilib>:"NT Write Number.vi"("Numeric"=w1166, "Name"=w1165) -> ()  [unwired: 9 in, 1 out]
      }
      event "Test Slider": Value Change {
        # "When the test mode slider helper is set, update that\ntree row item's value"
        n729 = event-data() -> ("NewVal"=w1172:dbl)  [unwired: 1 in]
        n730 = call <vilib>:"NT Write Number.vi"("Numeric"=w1172, "Name"=w1173) -> ()  [unwired: 9 in, 1 out]
      }
      event "On/Off": Value Change {
        # "When the test mode on/off helper value is set, update that\ntree row item's value"
        n731 = event-data() -> ("NewVal"=w1177:bool)  [unwired: 1 in]
        n732 = Boolean To (0,1)(Boolean=w1177) -> (0, 1=w1176:i16)
        n733 = call <vilib>:"NT Write Number.vi"("Numeric"=w1176, "Name"=w1175) -> ()  [unwired: 9 in, 1 out]
      }
      event "Rev/Fwd": Value Change {
        # "When the test mode helper value for relays is set, update that\ntree row item's value"
        n734 = event-data() -> ("NewVal.Forward"=w1185:bool, "NewVal.Reverse"=w1184:bool)  [unwired: 1 in]
        n735 = Boolean To (0,1)(Boolean=w1185) -> (0, 1=w1181:i16)
        n736 = Boolean To (0,1)(Boolean=w1184) -> (0, 1=w1183:i16)
        n737 = Negate(x=w1183) -> (-x=w1182:i16)
        n738 = Add(x=w1181, y=w1182) -> (x+y=w1180:i16)
        n739 = call <vilib>:"NT Write Number.vi"("Numeric"=w1180, "Name"=w1179) -> ()  [unwired: 9 in, 1 out]
      }
      event "Test Ring": Value Change {
        # "When a test mode helper value is selected from the ring,\nset the tree item's variable to the string value"
        n740 = event-data() -> ("NewVal"=w1189:u16)  [unwired: 1 in]
        n741 = property on="Test Ring" class="Ring (strict)"() -> ("Strings []"=w1190:string[])  [unwired: 2 in, 2 out]
        n742 = Index Array(array=w1190, index=w1189) -> (element=w1188:string)
        n743 = call <vilib>:"NT Write String.vi"("String"=w1188, "Name"=w1187) -> ()  [unwired: 9 in, 1 out]
      }
      event "Rec Mode": Value Change {
        # "Update globals for recording mode and path to read log from.\nClear when logging and let NetworkTables set path for vision to\nuse."
        n744 = event-data() -> ("NewVal"=w1199:enum32{"Stop", "Record", "Playback"})  [unwired: 1 in]
        n745 = global write "WPI_DashboardLogging Global.vi" "Logging Filename"(path "") -> ()
        n746 = global write "WPI_DashboardLogging Global.vi" "Recording"(w1199) -> ()
        n747 = case shown="\"Playback\"" w1199 {
          tunnel: w1198 -> [_ w1201 w1210]
          tunnel: [_ _ w1209] -> w1196
          tunnel: [_ _ w1208] -> _
          tunnel: w1194 -> [_ _ w1206]
          tunnel: cluster{i32, i32} {-250, 170} -> [_ _ w1205]
          tunnel: [_ _ T26 {"Image Size"=TRUE, "Image Type"=TRUE, "Pixel Value"=TRUE, "ROI Information"=TRUE, "Zoom Factor"=FALSE} ("Image Information Shown:All Elements")] -> _
          tunnel: [_ _ TRUE ("Zoom Factor")] -> _
          tunnel: w1192 -> [_ _ w1202]
          frame Default {
          }
          frame "Stop", "Record" {
            # "Place Window too"
            n748 = invoke class="VI" method="FP.Close"(reference=w1201) -> (reference out=w1200:refnum<vi>)  [unwired: 2 in, 2 out]
            n749 = invoke class="VI" method="Abort VI"(reference=w1200) -> ()  [unwired: 2 in, 3 out]
          }
          frame "Playback" {
            n750 = call "Open Playback Panel.vi"("Offset"=w1205, "DB VI Ref"=w1206, "Playback in"=w1210) -> ("Playback out"=w1207:refnum<vi>)  [unwired: 8 in]
            n751 = register-events(w1207, w1202) -> (reference out=w1209:refnum<event-registration>, error out=w1208:errorcluster)  [unwired: 2 in]
          }
        }
        n752 = call <vilib>:"WPI_DashboardNT Log FieldName Cache.vi"("Operation"=enum16{"Lookup/Add", "Index", "Clear"}."Clear") -> ()  [unwired: 8 in, 3 out]
      }
      event Panel Close {
        w1212 = enum32{"Stop", "Record", "Playback"}."Stop" ("Rec Mode")
        # "Playback window has been closed, abort"
        n753 = event-data() -> ()  [unwired: 1 in, 4 out]
        n754 = local write "Rec Mode"(w1212) -> ()
        n755 = global write "WPI_DashboardLogging Global.vi" "Recording"(w1212) -> ()
      }
      event Panel Close {
        # "Abort playback window and ourself"
        n756 = event-data() -> ()  [unwired: 1 in, 4 out]
        n757 = invoke class="VI" method="FP.Close"(reference=w1216) -> (reference out=w1215:refnum<vi>)  [unwired: 2 in, 2 out]
        n758 = invoke class="VI" method="Abort VI"(reference=w1215) -> (error out=w1214:errorcluster)  [unwired: 2 in, 2 out]
        n759 = invoke class="VI" method="Abort VI"(error in=w1214) -> ()  [unwired: 2 in, 3 out]
      }
      event User Event {
        n760 = event-data() -> ("IDs"=w1223:cluster{"RPC field ID":u16, "Unique ID":u16}, "String"=w1222:string)  [unwired: 1 in]
        n761 = Bundle("IDs"=w1223, "String"=w1222) -> (w1221:T11)  [unwired: 1 in]
        n762 = call <vilib>:"Retrieve RPC Response.vi"("RPC Response"=w1221) -> ("Output"=w1219:string[][])  [unwired: 10 in]
        n763 = Build Array (concatenate)(w1217, w1219) -> (w1218:string[][])
        n764 = local write "Command Params"(w1218) -> ()
        n765 = local write "Cmd Status"("" ("Cmd Status")) -> ()
      }
      event "Tree": Double Click {
        n766 = event-data() -> ("PlatMods"=w1229:T29, "Tag"=w1226:string)  [unwired: 1 in]
        n767 = Unbundle(w1229) -> ("Shift"=w1228:bool)  [unwired: 4 out]
        n768 = String Subset(string=w1226, length (rest)=1 ("length (rest)")) -> (substring=w1225:string)  [unwired: 1 in]
        n769 = Not(x=w1228) -> (.not. x?=w1227:bool)
        n770 = case shown="\"/\"" w1225 {
          tunnel: w1226 -> [_ w1232]
          tunnel: w1227 -> [_ w1231]
          frame Default {
          }
          frame "/" {
            n771 = call <vilib>:"NT Update Persistence.vi"("Persistence"=w1231, "Name"=w1232) -> ()  [unwired: 9 in, 1 out]
          }
        }
      }
    }
  }
  n772 = local write "Dashboard Tab"(T1."Setup/Auto" ("Dashboard Tab")) -> ()
  n773 = property class="VI"() -> ("Panel"=w35:refnum<vi>)  [unwired: 2 in, 2 out]
  n774 = property class="Pnl"(reference=w35) -> ("Panes[]"=w36:refnum<vi>[])  [unwired: 1 in, 2 out]
  n775 = property on="On/Off" class="Bool (strict)"("Visible"=w23) -> ()  [unwired: 2 in, 2 out]
  n776 = property on="Motor" class="Clust (strict)"("Visible"=w23) -> ()  [unwired: 2 in, 2 out]
  n777 = property on="Progress" class="Clust (strict)"("Visible"=w23) -> ()  [unwired: 2 in, 2 out]
  n778 = property on="Test Ring" class="Ring (strict)"("Visible"=w23) -> ()  [unwired: 2 in, 2 out]
  n779 = property on="Rev/Fwd" class="Clust (strict)"("Visible"=w23) -> ()  [unwired: 2 in, 2 out]
  n780 = Index Array(array=w36) -> (element=w34:refnum<vi>)  [unwired: 1 in]
  n781 = while {
    tunnel: w34 -> [w1234]
    i -> [w1237]
    stop <- FALSE stop-if-true
    n782 = Wait (ms)(milliseconds to wait=u32 100) -> ()  [unwired: 1 out]
    n783 = case shown="\"Playback\"" "Rec Mode" {
      tunnel: w1237 -> [_ _ w1252]
      tunnel: [u32 2829099 ("Base Color") u32 11141120 ("Target Color") w1241] -> w1233
      frame "Stop", Default {
        # "Reset the color, extra updates don't cost much"
      }
      frame "Record" {
      }
      frame "Playback" {
        # "Playback"
        n784 = Quotient & Remainder(x=w1252, y=u32 50 ("milliseconds to wait")) -> (x-y*floor(x/y)=w1248:u32)  [unwired: 1 out]
        n785 = Divide(x=w1248, y=u32 50 ("milliseconds to wait")) -> (x/y=w1245:dbl)
        n786 = Multiply(x=6.283185307179586, y=w1245) -> (x*y=w1250:dbl)
        n787 = Sine(x=w1250) -> (sin(x)=w1249:dbl)
        n788 = Absolute Value(x=w1249) -> (abs(x)=w1242:dbl)
        n789 = call "Interpolate RGB Color.vi"("Proportion"=w1242, "Target Color"=u32 30976, "Base Color"=u32 2829099) -> ("Result Color"=w1241:u32)  [unwired: 8 in]
      }
    }
    n790 = property class="Pane"(reference=w1234, "PaneColor"=w1233) -> ()  [unwired: 1 in, 2 out]
  }
  n791 = while {
    tunnel: u16 1741 ("timeout ms (25000)") -> [w1254]
    stop <- FALSE stop-if-true
    n792 = TCP Create Listener(10:w1254) -> (0:w1253:errorcluster, 3:w1255:refnum<k5>)  [unwired: 4 in, 1 out]
    n793 = case shown="No Error" w1253 {
      selector: w1253 -> [w1257 _]
      tunnel: w1255 -> [w1258 _]
      frame No Error {
        n794 = while {
          tunnel: w1258 -> [w1261]
          tunnel: w1257 -> [w1260]
          stop <- FALSE stop-if-true
          n795 = TCP Wait On Listener(8:w1260, 11:w1261) -> (0:w1262:errorcluster, 4:w1263:refnum<k5>)  [unwired: 2 in, 3 out]
          n796 = local write "TCP"(w1263) -> ()
          n797 = case shown="No Error" w1262 {
            frame No Error {
            }
            frame Error {
              n798 = Wait (ms)(milliseconds to wait=u32 1000) -> ()  [unwired: 1 out]
            }
          }
        }
      }
      frame Error {
        n799 = Wait (ms)(milliseconds to wait=u32 1000) -> ()  [unwired: 1 out]
      }
    }
  }
  n800 = local write "Command Selection"(u16 0 ("milliseconds to wait")) -> ()
  n801 = local write "Command Params"(string[][] [] ("Command Params")) -> ()
  n802 = while {
    tunnel: w8 -> [_]
    stop <- FALSE stop-if-true
    # "Error Message Handling"
    n803 = property on="Actuator Testing" class="Ring (strict)"() -> ("RingText.Text"=w1293:string)  [unwired: 2 in, 2 out]
    n804 = local read "Master_Safety_Override_1"() -> (w1367:bool)
    n805 = local read "Master_Safety_Override_2"() -> (w1368:bool)
    n806 = local read "Arm_Calibrate_Joysticks"() -> (w1279:bool)
    n807 = Wait (ms)(milliseconds to wait=u32 200) -> ()  [unwired: 1 out]
    n808 = local read "Shooter_Motor_Failure"() -> (w1314:bool)
    n809 = local read "Drive_Train_Shifter"() -> (w1270:bool)
    n810 = local read "CAN_Bus_Fault"() -> (w1276:bool)
    n811 = local read "Drive_Train_Overheat"() -> (w1346:bool)
    n812 = Not Equal?(x=w1293, y="No_Test") -> (x != y?=w1300:bool)
    n813 = local read "Drive_Train_Azimuth"() -> (w1337:bool)
    n814 = call <vilib>:"Space Constant.vi"() -> ("String"=w1291:string)
    n815 = local read "Shooter_Overheat"() -> (w1322:bool)
    n816 = local read "Super_Test_Mode"() -> (w1356:bool)
    n817 = local read "Auto_Test_Mode"() -> (w1325:bool)
    n818 = local read "Intake_Overheat"() -> (w1306:bool)
    n819 = local read "Battery_Critical"() -> (w1353:bool)
    n820 = local read "Electrical_Fault"() -> (w1284:bool)
    n821 = local read "Out_Of_Range"() -> (w1310:bool)
    n822 = local read "Arm_Calibrate"() -> (w1333:bool)
    n823 = local read "Pressure_Vent"() -> (w1342:bool)
    n824 = local read "Arm_Climber"() -> (w1317:bool)
    n825 = Search and Replace String(input string=w1293, search string="_", replace string=w1291) -> (result string=w1294:string)  [unwired: 5 in, 3 out]
    n826 = local read "IMU_Failure"() -> (w1297:bool)
    n827 = local read "Match_End"() -> (w1288:bool)
    n828 = local read "Slow_Loop"() -> (w1349:bool)
    n829 = local read "Auto_Error"() -> (w1330:bool)
    n830 = Concatenate Strings("testing " ("string"), w1294) -> (w1303:string)
    n831 = And(x=w1367, y=w1368) -> (x .and. y?=w1358:bool)
    n832 = Bundle("swerve shifter failure, forced into low gear", "Drive_Train_Shifter"=w1270, 600.0) -> (w1269:cluster{string, "Drive_Train_Shifter":bool, dbl})  [unwired: 1 in]
    n833 = Bundle("safeties disengaged", w1358, 10.0) -> (w1362:cluster{string, bool, dbl})  [unwired: 1 in]
    n834 = Bundle("super test mode", "Super_Test_Mode"=w1356, 10.0) -> (w1361:cluster{string, "Super_Test_Mode":bool, dbl})  [unwired: 1 in]
    n835 = Bundle("battery low", "Battery_Critical"=w1353, 600.0) -> (w1360:cluster{string, "Battery_Critical":bool, dbl})  [unwired: 1 in]
    n836 = Bundle("control latency too high", "Slow_Loop"=w1349, 60.0) -> (w1350:cluster{string, "Slow_Loop":bool, dbl})  [unwired: 1 in]
    n837 = Bundle("drive train overheating", "Drive_Train_Overheat"=w1346, 60.0) -> (w1345:T30)  [unwired: 1 in]
    n838 = Bundle("pressure venting", "Pressure_Vent"=w1342, 600.0) -> (w1341:cluster{string, "Pressure_Vent":bool, dbl})  [unwired: 1 in]
    n839 = Bundle("swerve module failure", "Drive_Train_Azimuth"=w1337, 600.0) -> (w1338:cluster{string, "Drive_Train_Azimuth":bool, dbl})  [unwired: 1 in]
    n840 = Bundle("ready to calibrate swerve modules", "Arm_Calibrate"=w1333, 10.0) -> (w1334:cluster{string, "Arm_Calibrate":bool, dbl})  [unwired: 1 in]
    n841 = Bundle("autonomous play failure", "Auto_Error"=w1330, 10.0) -> (w1329:cluster{string, "Auto_Error":bool, dbl})  [unwired: 1 in]
    n842 = Bundle("autonomous test mode", "Auto_Test_Mode"=w1325, 10.0) -> (w1326:cluster{string, "Auto_Test_Mode":bool, dbl})  [unwired: 1 in]
    n843 = Bundle("shooter overheating", "Shooter_Overheat"=w1322, 60.0) -> (w1321:cluster{string, "Shooter_Overheat":bool, dbl})  [unwired: 1 in]
    n844 = Bundle("climber is armed", "Arm_Climber"=w1317, 10.0) -> (w1318:cluster{string, "Arm_Climber":bool, dbl})  [unwired: 1 in]
    n845 = Bundle("shooter motor failure", "Shooter_Motor_Failure"=w1314, 60.0) -> (w1313:T31)  [unwired: 1 in]
    n846 = Bundle("out of range", "Out_Of_Range"=w1310, 5.0) -> (w1309:cluster{string, "Out_Of_Range":bool, dbl})  [unwired: 1 in]
    n847 = Bundle("intake overheating", "Intake_Overheat"=w1306, 60.0) -> (w1305:cluster{string, "Intake_Overheat":bool, dbl})  [unwired: 1 in]
    n848 = Bundle(w1303, w1300, 10.0) -> (w1299:cluster{string, bool, dbl})  [unwired: 1 in]
    n849 = Bundle("IMU failure, auto targeting disabled", "IMU_Failure"=w1297, 600.0) -> (w1295:cluster{string, "IMU_Failure":bool, dbl})  [unwired: 1 in]
    n850 = Bundle("begin endgame", "Match_End"=w1288, 10.0) -> (w1287:cluster{string, "Match_End":bool, dbl})  [unwired: 1 in]
    n851 = Bundle("electrical bus fault, power down immediately", "Electrical_Fault"=w1284, 60.0) -> (w1283:cluster{string, "Electrical_Fault":bool, dbl})  [unwired: 1 in]
    n852 = Bundle("ready to calibrate joysticks, wait ten seconds after pressing calibrate", "Arm_Calibrate_Joysticks"=w1279, 10.0) -> (w1280:T32)  [unwired: 1 in]
    n853 = Bundle("CAN bus fault, check wiring", "CAN_Bus_Fault"=w1276, 60.0) -> (w1278:cluster{string, "CAN_Bus_Fault":bool, dbl})  [unwired: 1 in]
    n854 = local read "Audible_Warnings_Enabled"() -> (w1268:bool)
    n855 = Build Array(w1362, w1361, w1360, w1350, w1345, w1341, w1338, w1334, w1329, w1326, w1321, w1318, w1313, w1309, w1305, w1299, w1295, w1287, w1283, w1280, w1278, w1269) -> (w1359:T33)
    n856 = call "EdgeTrigger.vi"("Input Signal"=w1268) -> ("All Edge Trigger"=w1267:bool)  [unwired: 2 out]
    n857 = call "ErrorMessageBuilder.vi"("Errors"=w1359, "Reset Error History"=w1267) -> ("Combined Error String"=w1273:string)
    n858 = Not Equal?(x="", y=w1273) -> (x != y?=w1274:bool)
    n859 = Compound Arithmetic op=AND(w1268, w1274) -> (w1266:bool)
    n860 = case shown="True" w1266 {
      tunnel: w1273 -> [_ w1372]
      frame False {
      }
      frame True {
        n861 = call "TextToSpeech.vi"("Text To Be Spoken"=w1372) -> ()  [unwired: 9 in, 2 out]
      }
    }
    n862 = case shown="True" w1274 {
      tunnel: w1273 -> [_ w1371]
      frame False {
      }
      frame True {
        "Combined Error String" <- w1371
      }
    }
  }
  n863 = global write "WPI_DashboardLogging Global.vi" "Recording"(w28) -> ()
  n864 = local write "Rec Mode"(w28) -> ()
  n865 = call <vilib>:"NT Write String.vi"("String"="Select Auto", "Name"="Auto Selector") -> ()  [unwired: 9 in, 1 out]
  n866 = while {
    stop <- FALSE stop-if-true
    # "Set window properties"
    n867 = Not(x="Dock_Dashboard") -> (.not. x?=w1374:bool)
    n868 = First Call?() -> (First Call?: T/F=w1378:bool)
    n869 = Wait (ms)(milliseconds to wait=u32 10) -> ()  [unwired: 1 out]
    n870 = Compound Arithmetic op=OR(w1374, w1378) -> (w1376:bool)
    n871 = control-ref of="This VI"() -> (w1377:refnum<vi>)
    n872 = call "EdgeTrigger.vi"("Input Signal"=w1376) -> ("Falling Edge Trigger"=w1375:bool)  [unwired: 2 out]
    n873 = case shown="True" w1376 {
      tunnel: w1377 -> [w1383 w1390]
      tunnel: w1375 -> [w1381 _]
      frame False {
        n874 = case shown="True" w1381 {
          tunnel: T34 {"Left"=100, "Top"=100, "Right"=1390, "Bottom"=585} ("Front Panel Window:Window Bounds") -> [_ w1389]
          tunnel: w1383 -> [w1386 w1388]
          tunnel: [w1386 w1387] -> w1382
          frame False {
          }
          frame True {
            n875 = property class="VI"(reference=w1388, "Front Panel.WinBounds"=w1389) -> (reference out=w1387:refnum<vi>)  [unwired: 1 in, 1 out]
          }
        }
        n876 = property class="VI"(reference=w1382, "Front Panel.TitleBarVis"=TRUE ("Front Panel Window:Title Bar Visible")) -> ()  [unwired: 1 in, 2 out]
      }
      frame True {
        n877 = property class="VI"(reference=w1390, "Front Panel.WinBounds"=T34 {"Left"=0, "Top"=0, "Right"=1290, "Bottom"=485} ("Front Panel Window:Window Bounds"), "Front Panel.TitleBarVis"=FALSE ("Front Panel Window:Title Bar Visible")) -> ()  [unwired: 1 in, 2 out]
      }
    }
  }
